vi "runtime execution.vi"() -> (0 "error out":errorcluster)   [LabVIEW 2013, in "Shared Memory Tests.lvlib"]
doc: "Copyright 2016 National Instruments Corporation\n\nLicensed under the Apache License, Version 2.0 (the \"License\"); you may not use this file except in compliance with the License. You may obtain a copy of the License at http://www.apache.org/licenses/LICENSE-2.0\nUnless required by applicable law or agreed to in writing, software distributed under the License is distributed on an \"AS IS\" BASIS, WITHOUT WARRANTIES OR CONDITIONS OF ANY KIND, either express or implied. See the License for the specific language governing permissions and limitations under the License."
uses:
  Shared Memory Tests.lvlib
  module/execution/Shared Memory Runtime.lvclass
  <vilib>/NI/Tag Bus/table/data table.lvlib
  <vilib>/NI/Tag Bus/table/data polymorphs/write many/write Doubles.vi
  <vilib>/NI/Tag Bus/table/data polymorphs/write many/write Booleans.vi
  <vilib>/NI/Tag Bus/table/data polymorphs/write many/write I32s.vi
  <vilib>/NI/Tag Bus/table/data polymorphs/write many/write Singles.vi
  <vilib>/NI/Tag Bus/table/data polymorphs/write many/write I64s.vi
  <vilib>/NI/Tag Bus/table/data polymorphs/write many/write I16s.vi
  <vilib>/NI/Tag Bus/table/data polymorphs/write many/write I8s.vi
  <vilib>/NI/Tag Bus/table/data polymorphs/write many/write U64s.vi
  <vilib>/NI/Tag Bus/table/data polymorphs/write many/write U32s.vi
  <vilib>/NI/Tag Bus/table/data polymorphs/write many/write U16s.vi
  <vilib>/NI/Tag Bus/table/data polymorphs/write many/write U8s.vi
  <vilib>/NI/Tag Bus/table/data polymorphs/write many/write Strings.vi
  module/configuration/Shared Memory Configuration.lvclass
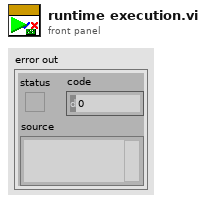
[diagram p1: front panel]
types:
  T1 = typedef "TBM channel.lvclass/data tables.ctl" = cluster{"input data":T2, "processing parameter":T2, "processing result":T2, "output data":T2}
  T2 = typedef "tag bus.lvlib/dictionary table pair.ctl" = cluster{"data dictionary":refnum<class "data dictionary.lvclass">, "data table":T3}
  T3 = typedef "tag bus.lvlib/data table.lvlib/data table.ctl" = cluster{"Double":dbl[], "Single":sgl[], "I64":i64[], "I32":i32[], "I16":i16[], "I8":i8[], "U64":u64[], "U32":u32[], "U16":u16[], "U8":u8[], "Boolean":bool[], "String":string[], "Array of Double":cluster{"DBL Array":dbl[]}[], "Array of Single":cluster{"SGL Array":sgl[]}[], "Array of I64":cluster{"I64 Array":i64[]}[], "Array of I32":cluster{"I32 Array":i32[]}[], "Array of I16":cluster{"I16 Array":i16[]}[], "Array of I8":cluster{"I8 Array":i8[]}[], "Array of U64":cluster{"U64 Array":u64[]}[], "Array of U32":cluster{"U32 Array":u32[]}[], "Array of U16":cluster{"U16 Array":u16[]}[], "Array of U8":cluster{"U8 Array":u8[]}[], "Array of Boolean":cluster{"Boolean Array":bool[]}[], "Array of String":cluster{"String Array":string[]}[]}
  T4 = typedef "current tag file io module runtime.lvclass/current tag file io configuration.ctl" = cluster{"refnum":refnum<file>, "name":string, "data type":T5, "number of tags":i32, "indices":cluster{"index":i32[]}, "data array":cluster{"data":dbl[]}, "file array":cluster{"data":dbl[]}}
  T5 = typedef "tag bus.lvlib/tag descriptor.lvclass/Data Type.ctl" = enum16{"Double", "Single", "I64", "I32", "I16", "I8", "U64", "U32", "U16", "U8", "Boolean", "String", "Array of Double", "Array of Single", "Array of I64", "Array of I32", "Array of I16", "Array of I8", "Array of U64", "Array of U32", "Array of U16", "Array of U8", "Array of Boolean", "Array of String"}
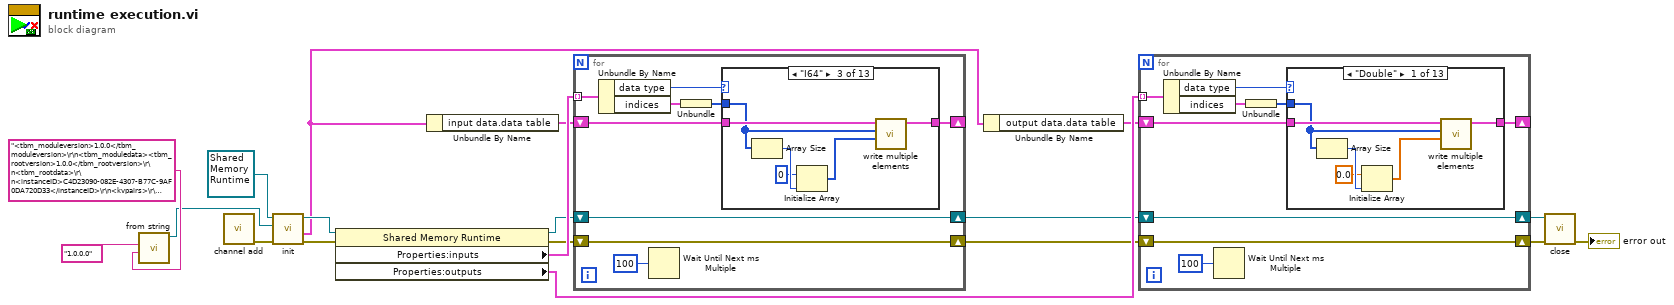
[diagram p0: block diagram]
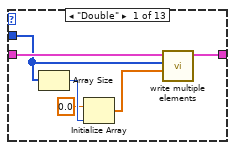
[diagram p2: hidden frame]
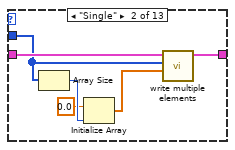
[diagram p3: hidden frame]
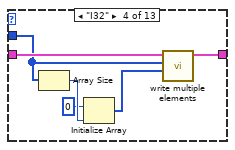
[diagram p4: hidden frame]
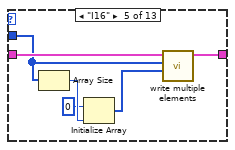
[diagram p5: hidden frame]
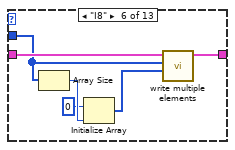
[diagram p6: hidden frame]
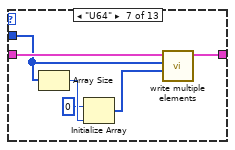
[diagram p7: hidden frame]
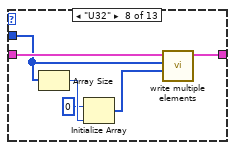
[diagram p8: hidden frame]
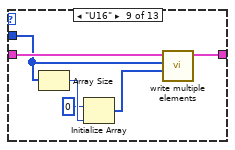
[diagram p9: hidden frame]
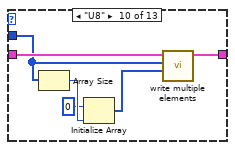
[diagram p10: hidden frame]
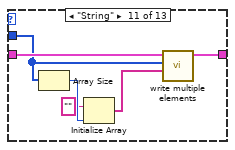
[diagram p11: hidden frame]
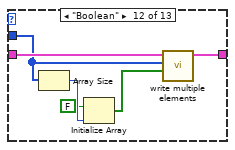
[diagram p12: hidden frame]
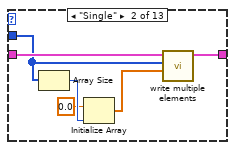
[diagram p14: hidden frame]
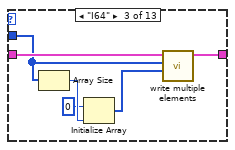
[diagram p15: hidden frame]
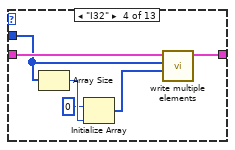
[diagram p16: hidden frame]
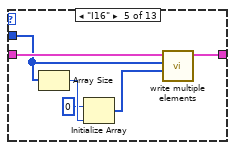
[diagram p17: hidden frame]
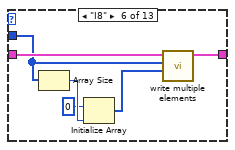
[diagram p18: hidden frame]
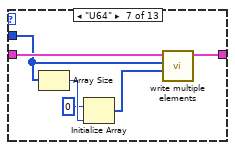
[diagram p19: hidden frame]
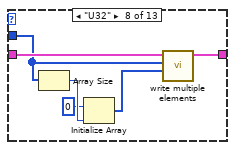
[diagram p20: hidden frame]
diagram:
  n1 = call-dynamic "from string.vi"("data"="<tbm_moduleversion>1.0.0</tbm_moduleversion>\r\n<tbm_moduledata><tbm_rootversion>1.0.0</tbm_rootversion>\r\n<tbm_rootdata>\r\n<instanceID>C4D23090-082E-4307-B77C-9AF0DA720D33</instanceID>\r\n<kvpairs>\r\n<SCFG_AliasName>Shared Memory</SCFG_AliasName>\r\n</kvpairs>\r\n</tbm_rootdata></tbm_moduledata>\r\n<Shared Memory><Cluster>\r\n<Name>shared memory configuration</Name>\r\n<NumElts>3</NumElts>\r\n<Array>\r\n<Name>lines</Name>\r\n<Dimsize>30</Dimsize>\r\n<Cluster>\r\n<Name>alarm config</Name>\r\n<NumElts>3</NumElts>\r\n<String>\r\n<Name>name</Name>\r\n<Val>AI0</Val>\r\n</String>\r\n<EW>\r\n<Name>data type</Name>\r\n<Choice>Double</Choice>\r\n<Choice>Single</Choice>\r\n<Choice>I64</Choice>\r\n<Choice>I32</Choice>\r\n<Choice>I16</Choice>\r\n<Choice>I8</Choice>\r\n<Choice>U64</Choice>\r\n<Choice>U32</Choice>\r\n<Choice>U16</Choice>\r\n<Choice>U8</Choice>\r\n<Choice>Boolean</Choice>\r\n<Choice>String</Choice>\r\n<Choice>Array of Double</Choice>\r\n<Choice>Array of Single</Choice>\r\n<Choice>Array of I64</Choice>\r\n<Choice>Array of I32</Choice>\r\n<Choice>Array of I16</Choice>\r\n<Choice>Array of I8</Choice>\r\n<Choice>Array of U64</Choice>\r\n<Choice>Array of U32</Choice>\r\n<Choice>Array of U16</Choice>\r\n<Choice>Array of U8</Choice>\r\n<Choice>Array of Boolean</Choice>\r\n<Choice>Array of String</Choice>\r\n<Val>0</Val>\r\n</EW>\r\n<Object>\r\n<Name>channel</Name>\r\n<NumLevels>2</NumLevels>\r\n<Class>TBM channel.lvclass</Class>\r\n<Version>1.0.0.3</Version>\r\n<Version>1.0.0.4</Version>\r\n<Cluster>\r\n<Name>tag descriptor.lvclass</Name>\r\n<NumElts>4</NumElts>\r\n<String>\r\n<Name>name</Name>\r\n<Val>AI0</Val>\r\n</String>\r\n<EW>\r\n<Name>data type</Name>\r\n<Choice>Double</Choice>\r\n<Choice>Single</Choice>\r\n<Choice>I64</Choice>\r\n<Choice>I32</Choice>\r\n<Choice>I16</Choice>\r\n<Choice>I8</Choice>\r\n<Choice>U64</Choice>\r\n<Choice>U32</Choice>\r\n<Choice>U16</Choice>\r\n<Choice>U8</Choice>\r\n<Choice>Boolean</Choice>\r\n<Choice>String</Choice>\r\n<Choice>Array of Double</Choice>\r\n<Choice>Array of Single</Choice>\r\n<Choice>Array of I64</Choice>\r\n<Choice>Array of I32</Choice>\r\n<Choice>Array of I16</Choice>\r\n<Choice>Array of I8</Choice>\r\n<Choice>Array of U64</Choice>\r\n<Choice>Array of U32</Choice>\r\n<Choice>Array of U16</Choice>\r\n<Choice>Array of U8</Choice>\r\n<Choice>Array of Boolean</Choice>\r\n<Choice>Array of String</Choice>\r\n<Val>0</Val>\r\n</EW>\r\n<String>\r\n<Name>default</Name>\r\n<Val></Val>\r\n</String>\r\n<String>\r\n<Name>metadata</Name>\r\n<Val></Val>\r\n</String>\r\n</Cluster>\r\n<Cluster>\r\n<Name>TBM channel.lvclass</Name>\r\n<NumElts>1</NumElts>\r\n<EW>\r\n<Name>channel classification</Name>\r\n<Choice>input data</Choice>\r\n<Choice>output data</Choice>\r\n<Choice>processing parameter</Choice>\r\n<Choice>processing result</Choice>\r\n<Val>1</Val>\r\n</EW>\r\n</Cluster>\r\n</Object>\r\n</Cluster>\r\n<Cluster>\r\n<Name>alarm config</Name>\r\n<NumElts>3</NumElts>\r\n<String>\r\n<Name>name</Name>\r\n<Val>AI1</Val>\r\n</String>\r\n<EW>\r\n<Name>data type</Name>\r\n<Choice>Double</Choice>\r\n<Choice>Single</Choice>\r\n<Choice>I64</Choice>\r\n<Choice>I32</Choice>\r\n<Choice>I16</Choice>\r\n<Choice>I8</Choice>\r\n<Choice>U64</Choice>\r\n<Choice>U32</Choice>\r\n<Choice>U16</Choice>\r\n<Choice>U8</Choice>\r\n<Choice>Boolean</Choice>\r\n<Choice>String</Choice>\r\n<Choice>Array of Double</Choice>\r\n<Choice>Array of Single</Choice>\r\n<Choice>Array of I64</Choice>\r\n<Choice>Array of I32</Choice>\r\n<Choice>Array of I16</Choice>\r\n<Choice>Array of I8</Choice>\r\n<Choice>Array of U64</Choice>\r\n<Choice>Array of U32</Choice>\r\n<Choice>Array of U16</Choice>\r\n<Choice>Array of U8</Choice>\r\n<Choice>Array of Boolean</Choice>\r\n<Choice>Array of String</Choice>\r\n<Val>10</Val>\r\n</EW>\r\n<Object>\r\n<Name>channel</Name>\r\n<NumLevels>2</NumLevels>\r\n<Class>TBM channel.lvclass</Class>\r\n<Version>1.0.0.3</Version>\r\n<Version>1.0.0.4</Version>\r\n<Cluster>\r\n<Name>tag descriptor.lvclass</Name>\r\n<NumElts>4</NumElts>\r\n<String>\r\n<Name>name</Name>\r\n<Val>AI1</Val>\r\n</String>\r\n<EW>\r\n<Name>data type</Name>\r\n<Choice>Double</Choice>\r\n<Choice>Single</Choice>\r\n<Choice>I64</Choice>\r\n<Choice>I32</Choice>\r\n<Choice>I16</Choice>\r\n<Choice>I8</Choice>\r\n<Choice>U64</Choice>\r\n<Choice>U32</Choice>\r\n<Choice>U16</Choice>\r\n<Choice>U8</Choice>\r\n<Choice>Boolean</Choice>\r\n<Choice>String</Choice>\r\n<Choice>Array of Double</Choice>\r\n<Choice>Array of Single</Choice>\r\n<Choice>Array of I64</Choice>\r\n<Choice>Array of I32</Choice>\r\n<Choice>Array of I16</Choice>\r\n<Choice>Array of I8</Choice>\r\n<Choice>Array of U64</Choice>\r\n<Choice>Array of U32</Choice>\r\n<Choice>Array of U16</Choice>\r\n<Choice>Array of U8</Choice>\r\n<Choice>Array of Boolean</Choice>\r\n<Choice>Array of String</Choice>\r\n<Val>10</Val>\r\n</EW>\r\n<String>\r\n<Name>default</Name>\r\n<Val></Val>\r\n</String>\r\n<String>\r\n<Name>metadata</Name>\r\n<Val></Val>\r\n</String>\r\n</Cluster>\r\n<Cluster>\r\n<Name>TBM channel.lvclass</Name>\r\n<NumElts>1</NumElts>\r\n<EW>\r\n<Name>channel classification</Name>\r\n<Choice>input data</Choice>\r\n<Choice>output data</Choice>\r\n<Choice>processing parameter</Choice>\r\n<Choice>processing result</Choice>\r\n<Val>1</Val>\r\n</EW>\r\n</Cluster>\r\n</Object>\r\n</Cluster>\r\n<Cluster>\r\n<Name>alarm config</Name>\r\n<NumElts>3</NumElts>\r\n<String>\r\n<Name>name</Name>\r\n<Val>AI2</Val>\r\n</String>\r\n<EW>\r\n<Name>data type</Name>\r\n<Choice>Double</Choice>\r\n<Choice>Single</Choice>\r\n<Choice>I64</Choice>\r\n<Choice>I32</Choice>\r\n<Choice>I16</Choice>\r\n<Choice>I8</Choice>\r\n<Choice>U64</Choice>\r\n<Choice>U32</Choice>\r\n<Choice>U16</Choice>\r\n<Choice>U8</Choice>\r\n<Choice>Boolean</Choice>\r\n<Choice>String</Choice>\r\n<Choice>Array of Double</Choice>\r\n<Choice>Array of Single</Choice>\r\n<Choice>Array of I64</Choice>\r\n<Choice>Array of I32</Choice>\r\n<Choice>Array of I16</Choice>\r\n<Choice>Array of I8</Choice>\r\n<Choice>Array of U64</Choice>\r\n<Choice>Array of U32</Choice>\r\n<Choice>Array of U16</Choice>\r\n<Choice>Array of U8</Choice>\r\n<Choice>Array of Boolean</Choice>\r\n<Choice>Array of String</Choice>\r\n<Val>3</Val>\r\n</EW>\r\n<Object>\r\n<Name>channel</Name>\r\n<NumLevels>2</NumLevels>\r\n<Class>TBM channel.lvclass</Class>\r\n<Version>1.0.0.3</Version>\r\n<Version>1.0.0.4</Version>\r\n<Cluster>\r\n<Name>tag descriptor.lvclass</Name>\r\n<NumElts>4</NumElts>\r\n<String>\r\n<Name>name</Name>\r\n<Val>AI2</Val>\r\n</String>\r\n<EW>\r\n<Name>data type</Name>\r\n<Choice>Double</Choice>\r\n<Choice>Single</Choice>\r\n<Choice>I64</Choice>\r\n<Choice>I32</Choice>\r\n<Choice>I16</Choice>\r\n<Choice>I8</Choice>\r\n<Choice>U64</Choice>\r\n<Choice>U32</Choice>\r\n<Choice>U16</Choice>\r\n<Choice>U8</Choice>\r\n<Choice>Boolean</Choice>\r\n<Choice>String</Choice>\r\n<Choice>Array of Double</Choice>\r\n<Choice>Array of Single</Choice>\r\n<Choice>Array of I64</Choice>\r\n<Choice>Array of I32</Choice>\r\n<Choice>Array of I16</Choice>\r\n<Choice>Array of I8</Choice>\r\n<Choice>Array of U64</Choice>\r\n<Choice>Array of U32</Choice>\r\n<Choice>Array of U16</Choice>\r\n<Choice>Array of U8</Choice>\r\n<Choice>Array of Boolean</Choice>\r\n<Choice>Array of String</Choice>\r\n<Val>3</Val>\r\n</EW>\r\n<String>\r\n<Name>default</Name>\r\n<Val></Val>\r\n</String>\r\n<String>\r\n<Name>metadata</Name>\r\n<Val></Val>\r\n</String>\r\n</Cluster>\r\n<Cluster>\r\n<Name>TBM channel.lvclass</Name>\r\n<NumElts>1</NumElts>\r\n<EW>\r\n<Name>channel classification</Name>\r\n<Choice>input data</Choice>\r\n<Choice>output data</Choice>\r\n<Choice>processing parameter</Choice>\r\n<Choice>processing result</Choice>\r\n<Val>1</Val>\r\n</EW>\r\n</Cluster>\r\n</Object>\r\n</Cluster>\r\n<Cluster>\r\n<Name>alarm config</Name>\r\n<NumElts>3</NumElts>\r\n<String>\r\n<Name>name</Name>\r\n<Val>AI3</Val>\r\n</String>\r\n<EW>\r\n<Name>data type</Name>\r\n<Choice>Double</Choice>\r\n<Choice>Single</Choice>\r\n<Choice>I64</Choice>\r\n<Choice>I32</Choice>\r\n<Choice>I16</Choice>\r\n<Choice>I8</Choice>\r\n<Choice>U64</Choice>\r\n<Choice>U32</Choice>\r\n<Choice>U16</Choice>\r\n<Choice>U8</Choice>\r\n<Choice>Boolean</Choice>\r\n<Choice>String</Choice>\r\n<Choice>Array of Double</Choice>\r\n<Choice>Array of Single</Choice>\r\n<Choice>Array of I64</Choice>\r\n<Choice>Array of I32</Choice>\r\n<Choice>Array of I16</Choice>\r\n<Choice>Array of I8</Choice>\r\n<Choice>Array of U64</Choice>\r\n<Choice>Array of U32</Choice>\r\n<Choice>Array of U16</Choice>\r\n<Choice>Array of U8</Choice>\r\n<Choice>Array of Boolean</Choice>\r\n<Choice>Array of String</Choice>\r\n<Val>0</Val>\r\n</EW>\r\n<Object>\r\n<Name>channel</Name>\r\n<NumLevels>2</NumLevels>\r\n<Class>TBM channel.lvclass</Class>\r\n<Version>1.0.0.3</Version>\r\n<Version>1.0.0.4</Version>\r\n<Cluster>\r\n<Name>tag descriptor.lvclass</Name>\r\n<NumElts>4</NumElts>\r\n<String>\r\n<Name>name</Name>\r\n<Val>AI3</Val>\r\n</String>\r\n<EW>\r\n<Name>data type</Name>\r\n<Choice>Double</Choice>\r\n<Choice>Single</Choice>\r\n<Choice>I64</Choice>\r\n<Choice>I32</Choice>\r\n<Choice>I16</Choice>\r\n<Choice>I8</Choice>\r\n<Choice>U64</Choice>\r\n<Choice>U32</Choice>\r\n<Choice>U16</Choice>\r\n<Choice>U8</Choice>\r\n<Choice>Boolean</Choice>\r\n<Choice>String</Choice>\r\n<Choice>Array of Double</Choice>\r\n<Choice>Array of Single</Choice>\r\n<Choice>Array of I64</Choice>\r\n<Choice>Array of I32</Choice>\r\n<Choice>Array of I16</Choice>\r\n<Choice>Array of I8</Choice>\r\n<Choice>Array of U64</Choice>\r\n<Choice>Array of U32</Choice>\r\n<Choice>Array of U16</Choice>\r\n<Choice>Array of U8</Choice>\r\n<Choice>Array of Boolean</Choice>\r\n<Choice>Array of String</Choice>\r\n<Val>0</Val>\r\n</EW>\r\n<String>\r\n<Name>default</Name>\r\n<Val></Val>\r\n</String>\r\n<String>\r\n<Name>metadata</Name>\r\n<Val></Val>\r\n</String>\r\n</Cluster>\r\n<Cluster>\r\n<Name>TBM channel.lvclass</Name>\r\n<NumElts>1</NumElts>\r\n<EW>\r\n<Name>channel classification</Name>\r\n<Choice>input data</Choice>\r\n<Choice>output data</Choice>\r\n<Choice>processing parameter</Choice>\r\n<Choice>processing result</Choice>\r\n<Val>1</Val>\r\n</EW>\r\n</Cluster>\r\n</Object>\r\n</Cluster>\r\n<Cluster>\r\n<Name>alarm config</Name>\r\n<NumElts>3</NumElts>\r\n<String>\r\n<Name>name</Name>\r\n<Val>AI4</Val>\r\n</String>\r\n<EW>\r\n<Name>data type</Name>\r\n<Choice>Double</Choice>\r\n<Choice>Single</Choice>\r\n<Choice>I64</Choice>\r\n<Choice>I32</Choice>\r\n<Choice>I16</Choice>\r\n<Choice>I8</Choice>\r\n<Choice>U64</Choice>\r\n<Choice>U32</Choice>\r\n<Choice>U16</Choice>\r\n<Choice>U8</Choice>\r\n<Choice>Boolean</Choice>\r\n<Choice>String</Choice>\r\n<Choice>Array of Double</Choice>\r\n<Choice>Array of Single</Choice>\r\n<Choice>Array of I64</Choice>\r\n<Choice>Array of I32</Choice>\r\n<Choice>Array of I16</Choice>\r\n<Choice>Array of I8</Choice>\r\n<Choice>Array of U64</Choice>\r\n<Choice>Array of U32</Choice>\r\n<Choice>Array of U16</Choice>\r\n<Choice>Array of U8</Choice>\r\n<Choice>Array of Boolean</Choice>\r\n<Choice>Array of String</Choice>\r\n<Val>10</Val>\r\n</EW>\r\n<Object>\r\n<Name>channel</Name>\r\n<NumLevels>2</NumLevels>\r\n<Class>TBM channel.lvclass</Class>\r\n<Version>1.0.0.3</Version>\r\n<Version>1.0.0.4</Version>\r\n<Cluster>\r\n<Name>tag descriptor.lvclass</Name>\r\n<NumElts>4</NumElts>\r\n<String>\r\n<Name>name</Name>\r\n<Val>AI4</Val>\r\n</String>\r\n<EW>\r\n<Name>data type</Name>\r\n<Choice>Double</Choice>\r\n<Choice>Single</Choice>\r\n<Choice>I64</Choice>\r\n<Choice>I32</Choice>\r\n<Choice>I16</Choice>\r\n<Choice>I8</Choice>\r\n<Choice>U64</Choice>\r\n<Choice>U32</Choice>\r\n<Choice>U16</Choice>\r\n<Choice>U8</Choice>\r\n<Choice>Boolean</Choice>\r\n<Choice>String</Choice>\r\n<Choice>Array of Double</Choice>\r\n<Choice>Array of Single</Choice>\r\n<Choice>Array of I64</Choice>\r\n<Choice>Array of I32</Choice>\r\n<Choice>Array of I16</Choice>\r\n<Choice>Array of I8</Choice>\r\n<Choice>Array of U64</Choice>\r\n<Choice>Array of U32</Choice>\r\n<Choice>Array of U16</Choice>\r\n<Choice>Array of U8</Choice>\r\n<Choice>Array of Boolean</Choice>\r\n<Choice>Array of String</Choice>\r\n<Val>10</Val>\r\n</EW>\r\n<String>\r\n<Name>default</Name>\r\n<Val></Val>\r\n</String>\r\n<String>\r\n<Name>metadata</Name>\r\n<Val></Val>\r\n</String>\r\n</Cluster>\r\n<Cluster>\r\n<Name>TBM channel.lvclass</Name>\r\n<NumElts>1</NumElts>\r\n<EW>\r\n<Name>channel classification</Name>\r\n<Choice>input data</Choice>\r\n<Choice>output data</Choice>\r\n<Choice>processing parameter</Choice>\r\n<Choice>processing result</Choice>\r\n<Val>1</Val>\r\n</EW>\r\n</Cluster>\r\n</Object>\r\n</Cluster>\r\n<Cluster>\r\n<Name>alarm config</Name>\r\n<NumElts>3</NumElts>\r\n<String>\r\n<Name>name</Name>\r\n<Val>AI5</Val>\r\n</String>\r\n<EW>\r\n<Name>data type</Name>\r\n<Choice>Double</Choice>\r\n<Choice>Single</Choice>\r\n<Choice>I64</Choice>\r\n<Choice>I32</Choice>\r\n<Choice>I16</Choice>\r\n<Choice>I8</Choice>\r\n<Choice>U64</Choice>\r\n<Choice>U32</Choice>\r\n<Choice>U16</Choice>\r\n<Choice>U8</Choice>\r\n<Choice>Boolean</Choice>\r\n<Choice>String</Choice>\r\n<Choice>Array of Double</Choice>\r\n<Choice>Array of Single</Choice>\r\n<Choice>Array of I64</Choice>\r\n<Choice>Array of I32</Choice>\r\n<Choice>Array of I16</Choice>\r\n<Choice>Array of I8</Choice>\r\n<Choice>Array of U64</Choice>\r\n<Choice>Array of U32</Choice>\r\n<Choice>Array of U16</Choice>\r\n<Choice>Array of U8</Choice>\r\n<Choice>Array of Boolean</Choice>\r\n<Choice>Array of String</Choice>\r\n<Val>3</Val>\r\n</EW>\r\n<Object>\r\n<Name>channel</Name>\r\n<NumLevels>2</NumLevels>\r\n<Class>TBM channel.lvclass</Class>\r\n<Version>1.0.0.3</Version>\r\n<Version>1.0.0.4</Version>\r\n<Cluster>\r\n<Name>tag descriptor.lvclass</Name>\r\n<NumElts>4</NumElts>\r\n<String>\r\n<Name>name</Name>\r\n<Val>AI5</Val>\r\n</String>\r\n<EW>\r\n<Name>data type</Name>\r\n<Choice>Double</Choice>\r\n<Choice>Single</Choice>\r\n<Choice>I64</Choice>\r\n<Choice>I32</Choice>\r\n<Choice>I16</Choice>\r\n<Choice>I8</Choice>\r\n<Choice>U64</Choice>\r\n<Choice>U32</Choice>\r\n<Choice>U16</Choice>\r\n<Choice>U8</Choice>\r\n<Choice>Boolean</Choice>\r\n<Choice>String</Choice>\r\n<Choice>Array of Double</Choice>\r\n<Choice>Array of Single</Choice>\r\n<Choice>Array of I64</Choice>\r\n<Choice>Array of I32</Choice>\r\n<Choice>Array of I16</Choice>\r\n<Choice>Array of I8</Choice>\r\n<Choice>Array of U64</Choice>\r\n<Choice>Array of U32</Choice>\r\n<Choice>Array of U16</Choice>\r\n<Choice>Array of U8</Choice>\r\n<Choice>Array of Boolean</Choice>\r\n<Choice>Array of String</Choice>\r\n<Val>3</Val>\r\n</EW>\r\n<String>\r\n<Name>default</Name>\r\n<Val></Val>\r\n</String>\r\n<String>\r\n<Name>metadata</Name>\r\n<Val></Val>\r\n</String>\r\n</Cluster>\r\n<Cluster>\r\n<Name>TBM channel.lvclass</Name>\r\n<NumElts>1</NumElts>\r\n<EW>\r\n<Name>channel classification</Name>\r\n<Choice>input data</Choice>\r\n<Choice>output data</Choice>\r\n<Choice>processing parameter</Choice>\r\n<Choice>processing result</Choice>\r\n<Val>1</Val>\r\n</EW>\r\n</Cluster>\r\n</Object>\r\n</Cluster>\r\n<Cluster>\r\n<Name>alarm config</Name>\r\n<NumElts>3</NumElts>\r\n<String>\r\n<Name>name</Name>\r\n<Val>AI6</Val>\r\n</String>\r\n<EW>\r\n<Name>data type</Name>\r\n<Choice>Double</Choice>\r\n<Choice>Single</Choice>\r\n<Choice>I64</Choice>\r\n<Choice>I32</Choice>\r\n<Choice>I16</Choice>\r\n<Choice>I8</Choice>\r\n<Choice>U64</Choice>\r\n<Choice>U32</Choice>\r\n<Choice>U16</Choice>\r\n<Choice>U8</Choice>\r\n<Choice>Boolean</Choice>\r\n<Choice>String</Choice>\r\n<Choice>Array of Double</Choice>\r\n<Choice>Array of Single</Choice>\r\n<Choice>Array of I64</Choice>\r\n<Choice>Array of I32</Choice>\r\n<Choice>Array of I16</Choice>\r\n<Choice>Array of I8</Choice>\r\n<Choice>Array of U64</Choice>\r\n<Choice>Array of U32</Choice>\r\n<Choice>Array of U16</Choice>\r\n<Choice>Array of U8</Choice>\r\n<Choice>Array of Boolean</Choice>\r\n<Choice>Array of String</Choice>\r\n<Val>0</Val>\r\n</EW>\r\n<Object>\r\n<Name>channel</Name>\r\n<NumLevels>2</NumLevels>\r\n<Class>TBM channel.lvclass</Class>\r\n<Version>1.0.0.3</Version>\r\n<Version>1.0.0.4</Version>\r\n<Cluster>\r\n<Name>tag descriptor.lvclass</Name>\r\n<NumElts>4</NumElts>\r\n<String>\r\n<Name>name</Name>\r\n<Val>AI6</Val>\r\n</String>\r\n<EW>\r\n<Name>data type</Name>\r\n<Choice>Double</Choice>\r\n<Choice>Single</Choice>\r\n<Choice>I64</Choice>\r\n<Choice>I32</Choice>\r\n<Choice>I16</Choice>\r\n<Choice>I8</Choice>\r\n<Choice>U64</Choice>\r\n<Choice>U32</Choice>\r\n<Choice>U16</Choice>\r\n<Choice>U8</Choice>\r\n<Choice>Boolean</Choice>\r\n<Choice>String</Choice>\r\n<Choice>Array of Double</Choice>\r\n<Choice>Array of Single</Choice>\r\n<Choice>Array of I64</Choice>\r\n<Choice>Array of I32</Choice>\r\n<Choice>Array of I16</Choice>\r\n<Choice>Array of I8</Choice>\r\n<Choice>Array of U64</Choice>\r\n<Choice>Array of U32</Choice>\r\n<Choice>Array of U16</Choice>\r\n<Choice>Array of U8</Choice>\r\n<Choice>Array of Boolean</Choice>\r\n<Choice>Array of String</Choice>\r\n<Val>0</Val>\r\n</EW>\r\n<String>\r\n<Name>default</Name>\r\n<Val></Val>\r\n</String>\r\n<String>\r\n<Name>metadata</Name>\r\n<Val></Val>\r\n</String>\r\n</Cluster>\r\n<Cluster>\r\n<Name>TBM channel.lvclass</Name>\r\n<NumElts>1</NumElts>\r\n<EW>\r\n<Name>channel classification</Name>\r\n<Choice>input data</Choice>\r\n<Choice>output data</Choice>\r\n<Choice>processing parameter</Choice>\r\n<Choice>processing result</Choice>\r\n<Val>1</Val>\r\n</EW>\r\n</Cluster>\r\n</Object>\r\n</Cluster>\r\n<Cluster>\r\n<Name>alarm config</Name>\r\n<NumElts>3</NumElts>\r\n<String>\r\n<Name>name</Name>\r\n<Val>AI7</Val>\r\n</String>\r\n<EW>\r\n<Name>data type</Name>\r\n<Choice>Double</Choice>\r\n<Choice>Single</Choice>\r\n<Choice>I64</Choice>\r\n<Choice>I32</Choice>\r\n<Choice>I16</Choice>\r\n<Choice>I8</Choice>\r\n<Choice>U64</Choice>\r\n<Choice>U32</Choice>\r\n<Choice>U16</Choice>\r\n<Choice>U8</Choice>\r\n<Choice>Boolean</Choice>\r\n<Choice>String</Choice>\r\n<Choice>Array of Double</Choice>\r\n<Choice>Array of Single</Choice>\r\n<Choice>Array of I64</Choice>\r\n<Choice>Array of I32</Choice>\r\n<Choice>Array of I16</Choice>\r\n<Choice>Array of I8</Choice>\r\n<Choice>Array of U64</Choice>\r\n<Choice>Array of U32</Choice>\r\n<Choice>Array of U16</Choice>\r\n<Choice>Array of U8</Choice>\r\n<Choice>Array of Boolean</Choice>\r\n<Choice>Array of String</Choice>\r\n<Val>10</Val>\r\n</EW>\r\n<Object>\r\n<Name>channel</Name>\r\n<NumLevels>2</NumLevels>\r\n<Class>TBM channel.lvclass</Class>\r\n<Version>1.0.0.3</Version>\r\n<Version>1.0.0.4</Version>\r\n<Cluster>\r\n<Name>tag descriptor.lvclass</Name>\r\n<NumElts>4</NumElts>\r\n<String>\r\n<Name>name</Name>\r\n<Val>AI7</Val>\r\n</String>\r\n<EW>\r\n<Name>data type</Name>\r\n<Choice>Double</Choice>\r\n<Choice>Single</Choice>\r\n<Choice>I64</Choice>\r\n<Choice>I32</Choice>\r\n<Choice>I16</Choice>\r\n<Choice>I8</Choice>\r\n<Choice>U64</Choice>\r\n<Choice>U32</Choice>\r\n<Choice>U16</Choice>\r\n<Choice>U8</Choice>\r\n<Choice>Boolean</Choice>\r\n<Choice>String</Choice>\r\n<Choice>Array of Double</Choice>\r\n<Choice>Array of Single</Choice>\r\n<Choice>Array of I64</Choice>\r\n<Choice>Array of I32</Choice>\r\n<Choice>Array of I16</Choice>\r\n<Choice>Array of I8</Choice>\r\n<Choice>Array of U64</Choice>\r\n<Choice>Array of U32</Choice>\r\n<Choice>Array of U16</Choice>\r\n<Choice>Array of U8</Choice>\r\n<Choice>Array of Boolean</Choice>\r\n<Choice>Array of String</Choice>\r\n<Val>10</Val>\r\n</EW>\r\n<String>\r\n<Name>default</Name>\r\n<Val></Val>\r\n</String>\r\n<String>\r\n<Name>metadata</Name>\r\n<Val></Val>\r\n</String>\r\n</Cluster>\r\n<Cluster>\r\n<Name>TBM channel.lvclass</Name>\r\n<NumElts>1</NumElts>\r\n<EW>\r\n<Name>channel classification</Name>\r\n<Choice>input data</Choice>\r\n<Choice>output data</Choice>\r\n<Choice>processing parameter</Choice>\r\n<Choice>processing result</Choice>\r\n<Val>1</Val>\r\n</EW>\r\n</Cluster>\r\n</Object>\r\n</Cluster>\r\n<Cluster>\r\n<Name>alarm config</Name>\r\n<NumElts>3</NumElts>\r\n<String>\r\n<Name>name</Name>\r\n<Val>AI8</Val>\r\n</String>\r\n<EW>\r\n<Name>data type</Name>\r\n<Choice>Double</Choice>\r\n<Choice>Single</Choice>\r\n<Choice>I64</Choice>\r\n<Choice>I32</Choice>\r\n<Choice>I16</Choice>\r\n<Choice>I8</Choice>\r\n<Choice>U64</Choice>\r\n<Choice>U32</Choice>\r\n<Choice>U16</Choice>\r\n<Choice>U8</Choice>\r\n<Choice>Boolean</Choice>\r\n<Choice>String</Choice>\r\n<Choice>Array of Double</Choice>\r\n<Choice>Array of Single</Choice>\r\n<Choice>Array of I64</Choice>\r\n<Choice>Array of I32</Choice>\r\n<Choice>Array of I16</Choice>\r\n<Choice>Array of I8</Choice>\r\n<Choice>Array of U64</Choice>\r\n<Choice>Array of U32</Choice>\r\n<Choice>Array of U16</Choice>\r\n<Choice>Array of U8</Choice>\r\n<Choice>Array of Boolean</Choice>\r\n<Choice>Array of String</Choice>\r\n<Val>3</Val>\r\n</EW>\r\n<Object>\r\n<Name>channel</Name>\r\n<NumLevels>2</NumLevels>\r\n<Class>TBM channel.lvclass</Class>\r\n<Version>1.0.0.3</Version>\r\n<Version>1.0.0.4</Version>\r\n<Cluster>\r\n<Name>tag descriptor.lvclass</Name>\r\n<NumElts>4</NumElts>\r\n<String>\r\n<Name>name</Name>\r\n<Val>AI8</Val>\r\n</String>\r\n<EW>\r\n<Name>data type</Name>\r\n<Choice>Double</Choice>\r\n<Choice>Single</Choice>\r\n<Choice>I64</Choice>\r\n<Choice>I32</Choice>\r\n<Choice>I16</Choice>\r\n<Choice>I8</Choice>\r\n<Choice>U64</Choice>\r\n<Choice>U32</Choice>\r\n<Choice>U16</Choice>\r\n<Choice>U8</Choice>\r\n<Choice>Boolean</Choice>\r\n<Choice>String</Choice>\r\n<Choice>Array of Double</Choice>\r\n<Choice>Array of Single</Choice>\r\n<Choice>Array of I64</Choice>\r\n<Choice>Array of I32</Choice>\r\n<Choice>Array of I16</Choice>\r\n<Choice>Array of I8</Choice>\r\n<Choice>Array of U64</Choice>\r\n<Choice>Array of U32</Choice>\r\n<Choice>Array of U16</Choice>\r\n<Choice>Array of U8</Choice>\r\n<Choice>Array of Boolean</Choice>\r\n<Choice>Array of String</Choice>\r\n<Val>3</Val>\r\n</EW>\r\n<String>\r\n<Name>default</Name>\r\n<Val></Val>\r\n</String>\r\n<String>\r\n<Name>metadata</Name>\r\n<Val></Val>\r\n</String>\r\n</Cluster>\r\n<Cluster>\r\n<Name>TBM channel.lvclass</Name>\r\n<NumElts>1</NumElts>\r\n<EW>\r\n<Name>channel classification</Name>\r\n<Choice>input data</Choice>\r\n<Choice>output data</Choice>\r\n<Choice>processing parameter</Choice>\r\n<Choice>processing result</Choice>\r\n<Val>1</Val>\r\n</EW>\r\n</Cluster>\r\n</Object>\r\n</Cluster>\r\n<Cluster>\r\n<Name>alarm config</Name>\r\n<NumElts>3</NumElts>\r\n<String>\r\n<Name>name</Name>\r\n<Val>AI9</Val>\r\n</String>\r\n<EW>\r\n<Name>data type</Name>\r\n<Choice>Double</Choice>\r\n<Choice>Single</Choice>\r\n<Choice>I64</Choice>\r\n<Choice>I32</Choice>\r\n<Choice>I16</Choice>\r\n<Choice>I8</Choice>\r\n<Choice>U64</Choice>\r\n<Choice>U32</Choice>\r\n<Choice>U16</Choice>\r\n<Choice>U8</Choice>\r\n<Choice>Boolean</Choice>\r\n<Choice>String</Choice>\r\n<Choice>Array of Double</Choice>\r\n<Choice>Array of Single</Choice>\r\n<Choice>Array of I64</Choice>\r\n<Choice>Array of I32</Choice>\r\n<Choice>Array of I16</Choice>\r\n<Choice>Array of I8</Choice>\r\n<Choice>Array of U64</Choice>\r\n<Choice>Array of U32</Choice>\r\n<Choice>Array of U16</Choice>\r\n<Choice>Array of U8</Choice>\r\n<Choice>Array of Boolean</Choice>\r\n<Choice>Array of String</Choice>\r\n<Val>0</Val>\r\n</EW>\r\n<Object>\r\n<Name>channel</Name>\r\n<NumLevels>2</NumLevels>\r\n<Class>TBM channel.lvclass</Class>\r\n<Version>1.0.0.3</Version>\r\n<Version>1.0.0.4</Version>\r\n<Cluster>\r\n<Name>tag descriptor.lvclass</Name>\r\n<NumElts>4</NumElts>\r\n<String>\r\n<Name>name</Name>\r\n<Val>AI9</Val>\r\n</String>\r\n<EW>\r\n<Name>data type</Name>\r\n<Choice>Double</Choice>\r\n<Choice>Single</Choice>\r\n<Choice>I64</Choice>\r\n<Choice>I32</Choice>\r\n<Choice>I16</Choice>\r\n<Choice>I8</Choice>\r\n<Choice>U64</Choice>\r\n<Choice>U32</Choice>\r\n<Choice>U16</Choice>\r\n<Choice>U8</Choice>\r\n<Choice>Boolean</Choice>\r\n<Choice>String</Choice>\r\n<Choice>Array of Double</Choice>\r\n<Choice>Array of Single</Choice>\r\n<Choice>Array of I64</Choice>\r\n<Choice>Array of I32</Choice>\r\n<Choice>Array of I16</Choice>\r\n<Choice>Array of I8</Choice>\r\n<Choice>Array of U64</Choice>\r\n<Choice>Array of U32</Choice>\r\n<Choice>Array of U16</Choice>\r\n<Choice>Array of U8</Choice>\r\n<Choice>Array of Boolean</Choice>\r\n<Choice>Array of String</Choice>\r\n<Val>0</Val>\r\n</EW>\r\n<String>\r\n<Name>default</Name>\r\n<Val></Val>\r\n</String>\r\n<String>\r\n<Name>metadata</Name>\r\n<Val></Val>\r\n</String>\r\n</Cluster>\r\n<Cluster>\r\n<Name>TBM channel.lvclass</Name>\r\n<NumElts>1</NumElts>\r\n<EW>\r\n<Name>channel classification</Name>\r\n<Choice>input data</Choice>\r\n<Choice>output data</Choice>\r\n<Choice>processing parameter</Choice>\r\n<Choice>processing result</Choice>\r\n<Val>1</Val>\r\n</EW>\r\n</Cluster>\r\n</Object>\r\n</Cluster>\r\n<Cluster>\r\n<Name>alarm config</Name>\r\n<NumElts>3</NumElts>\r\n<String>\r\n<Name>name</Name>\r\n<Val>AO0</Val>\r\n</String>\r\n<EW>\r\n<Name>data type</Name>\r\n<Choice>Double</Choice>\r\n<Choice>Single</Choice>\r\n<Choice>I64</Choice>\r\n<Choice>I32</Choice>\r\n<Choice>I16</Choice>\r\n<Choice>I8</Choice>\r\n<Choice>U64</Choice>\r\n<Choice>U32</Choice>\r\n<Choice>U16</Choice>\r\n<Choice>U8</Choice>\r\n<Choice>Boolean</Choice>\r\n<Choice>String</Choice>\r\n<Choice>Array of Double</Choice>\r\n<Choice>Array of Single</Choice>\r\n<Choice>Array of I64</Choice>\r\n<Choice>Array of I32</Choice>\r\n<Choice>Array of I16</Choice>\r\n<Choice>Array of I8</Choice>\r\n<Choice>Array of U64</Choice>\r\n<Choice>Array of U32</Choice>\r\n<Choice>Array of U16</Choice>\r\n<Choice>Array of U8</Choice>\r\n<Choice>Array of Boolean</Choice>\r\n<Choice>Array of String</Choice>\r\n<Val>10</Val>\r\n</EW>\r\n<Object>\r\n<Name>channel</Name>\r\n<NumLevels>2</NumLevels>\r\n<Class>TBM channel.lvclass</Class>\r\n<Version>1.0.0.3</Version>\r\n<Version>1.0.0.4</Version>\r\n<Cluster>\r\n<Name>tag descriptor.lvclass</Name>\r\n<NumElts>4</NumElts>\r\n<String>\r\n<Name>name</Name>\r\n<Val>AO0</Val>\r\n</String>\r\n<EW>\r\n<Name>data type</Name>\r\n<Choice>Double</Choice>\r\n<Choice>Single</Choice>\r\n<Choice>I64</Choice>\r\n<Choice>I32</Choice>\r\n<Choice>I16</Choice>\r\n<Choice>I8</Choice>\r\n<Choice>U64</Choice>\r\n<Choice>U32</Choice>\r\n<Choice>U16</Choice>\r\n<Choice>U8</Choice>\r\n<Choice>Boolean</Choice>\r\n<Choice>String</Choice>\r\n<Choice>Array of Double</Choice>\r\n<Choice>Array of Single</Choice>\r\n<Choice>Array of I64</Choice>\r\n<Choice>Array of I32</Choice>\r\n<Choice>Array of I16</Choice>\r\n<Choice>Array of I8</Choice>\r\n<Choice>Array of U64</Choice>\r\n<Choice>Array of U32</Choice>\r\n<Choice>Array of U16</Choice>\r\n<Choice>Array of U8</Choice>\r\n<Choice>Array of Boolean</Choice>\r\n<Choice>Array of String</Choice>\r\n<Val>10</Val>\r\n</EW>\r\n<String>\r\n<Name>default</Name>\r\n<Val></Val>\r\n</String>\r\n<String>\r\n<Name>metadata</Name>\r\n<Val></Val>\r\n</String>\r\n</Cluster>\r\n<Cluster>\r\n</Cluster>\r\n</Object>\r\n</Cluster>\r\n<Cluster>\r\n<Name>alarm config</Name>\r\n<NumElts>3</NumElts>\r\n<String>\r\n<Name>name</Name>\r\n<Val>AO1</Val>\r\n</String>\r\n<EW>\r\n<Name>data type</Name>\r\n<Choice>Double</Choice>\r\n<Choice>Single</Choice>\r\n<Choice>I64</Choice>\r\n<Choice>I32</Choice>\r\n<Choice>I16</Choice>\r\n<Choice>I8</Choice>\r\n<Choice>U64</Choice>\r\n<Choice>U32</Choice>\r\n<Choice>U16</Choice>\r\n<Choice>U8</Choice>\r\n<Choice>Boolean</Choice>\r\n<Choice>String</Choice>\r\n<Choice>Array of Double</Choice>\r\n<Choice>Array of Single</Choice>\r\n<Choice>Array of I64</Choice>\r\n<Choice>Array of I32</Choice>\r\n<Choice>Array of I16</Choice>\r\n<Choice>Array of I8</Choice>\r\n<Choice>Array of U64</Choice>\r\n<Choice>Array of U32</Choice>\r\n<Choice>Array of U16</Choice>\r\n<Choice>Array of U8</Choice>\r\n<Choice>Array of Boolean</Choice>\r\n<Choice>Array of String</Choice>\r\n<Val>3</Val>\r\n</EW>\r\n<Object>\r\n<Name>channel</Name>\r\n<NumLevels>2</NumLevels>\r\n<Class>TBM channel.lvclass</Class>\r\n<Version>1.0.0.3</Version>\r\n<Version>1.0.0.4</Version>\r\n<Cluster>\r\n<Name>tag descriptor.lvclass</Name>\r\n<NumElts>4</NumElts>\r\n<String>\r\n<Name>name</Name>\r\n<Val>AO1</Val>\r\n</String>\r\n<EW>\r\n<Name>data type</Name>\r\n<Choice>Double</Choice>\r\n<Choice>Single</Choice>\r\n<Choice>I64</Choice>\r\n<Choice>I32</Choice>\r\n<Choice>I16</Choice>\r\n<Choice>I8</Choice>\r\n<Choice>U64</Choice>\r\n<Choice>U32</Choice>\r\n<Choice>U16</Choice>\r\n<Choice>U8</Choice>\r\n<Choice>Boolean</Choice>\r\n<Choice>String</Choice>\r\n<Choice>Array of Double</Choice>\r\n<Choice>Array of Single</Choice>\r\n<Choice>Array of I64</Choice>\r\n<Choice>Array of I32</Choice>\r\n<Choice>Array of I16</Choice>\r\n<Choice>Array of I8</Choice>\r\n<Choice>Array of U64</Choice>\r\n<Choice>Array of U32</Choice>\r\n<Choice>Array of U16</Choice>\r\n<Choice>Array of U8</Choice>\r\n<Choice>Array of Boolean</Choice>\r\n<Choice>Array of String</Choice>\r\n<Val>3</Val>\r\n</EW>\r\n<String>\r\n<Name>default</Name>\r\n<Val></Val>\r\n</String>\r\n<String>\r\n<Name>metadata</Name>\r\n<Val></Val>\r\n</String>\r\n</Cluster>\r\n<Cluster>\r\n</Cluster>\r\n</Object>\r\n</Cluster>\r\n<Cluster>\r\n<Name>alarm config</Name>\r\n<NumElts>3</NumElts>\r\n<String>\r\n<Name>name</Name>\r\n<Val>AO2</Val>\r\n</String>\r\n<EW>\r\n<Name>data type</Name>\r\n<Choice>Double</Choice>\r\n<Choice>Single</Choice>\r\n<Choice>I64</Choice>\r\n<Choice>I32</Choice>\r\n<Choice>I16</Choice>\r\n<Choice>I8</Choice>\r\n<Choice>U64</Choice>\r\n<Choice>U32</Choice>\r\n<Choice>U16</Choice>\r\n<Choice>U8</Choice>\r\n<Choice>Boolean</Choice>\r\n<Choice>String</Choice>\r\n<Choice>Array of Double</Choice>\r\n<Choice>Array of Single</Choice>\r\n<Choice>Array of I64</Choice>\r\n<Choice>Array of I32</Choice>\r\n<Choice>Array of I16</Choice>\r\n<Choice>Array of I8</Choice>\r\n<Choice>Array of U64</Choice>\r\n<Choice>Array of U32</Choice>\r\n<Choice>Array of U16</Choice>\r\n<Choice>Array of U8</Choice>\r\n<Choice>Array of Boolean</Choice>\r\n<Choice>Array of String</Choice>\r\n<Val>0</Val>\r\n</EW>\r\n<Object>\r\n<Name>channel</Name>\r\n<NumLevels>2</NumLevels>\r\n<Class>TBM channel.lvclass</Class>\r\n<Version>1.0.0.3</Version>\r\n<Version>1.0.0.4</Version>\r\n<Cluster>\r\n<Name>tag descriptor.lvclass</Name>\r\n<NumElts>4</NumElts>\r\n<String>\r\n<Name>name</Name>\r\n<Val>AO2</Val>\r\n</String>\r\n<EW>\r\n<Name>data type</Name>\r\n<Choice>Double</Choice>\r\n<Choice>Single</Choice>\r\n<Choice>I64</Choice>\r\n<Choice>I32</Choice>\r\n<Choice>I16</Choice>\r\n<Choice>I8</Choice>\r\n<Choice>U64</Choice>\r\n<Choice>U32</Choice>\r\n<Choice>U16</Choice>\r\n<Choice>U8</Choice>\r\n<Choice>Boolean</Choice>\r\n<Choice>String</Choice>\r\n<Choice>Array of Double</Choice>\r\n<Choice>Array of Single</Choice>\r\n<Choice>Array of I64</Choice>\r\n<Choice>Array of I32</Choice>\r\n<Choice>Array of I16</Choice>\r\n<Choice>Array of I8</Choice>\r\n<Choice>Array of U64</Choice>\r\n<Choice>Array of U32</Choice>\r\n<Choice>Array of U16</Choice>\r\n<Choice>Array of U8</Choice>\r\n<Choice>Array of Boolean</Choice>\r\n<Choice>Array of String</Choice>\r\n<Val>0</Val>\r\n</EW>\r\n<String>\r\n<Name>default</Name>\r\n<Val></Val>\r\n</String>\r\n<String>\r\n<Name>metadata</Name>\r\n<Val></Val>\r\n</String>\r\n</Cluster>\r\n<Cluster>\r\n</Cluster>\r\n</Object>\r\n</Cluster>\r\n<Cluster>\r\n<Name>alarm config</Name>\r\n<NumElts>3</NumElts>\r\n<String>\r\n<Name>name</Name>\r\n<Val>AO3</Val>\r\n</String>\r\n<EW>\r\n<Name>data type</Name>\r\n<Choice>Double</Choice>\r\n<Choice>Single</Choice>\r\n<Choice>I64</Choice>\r\n<Choice>I32</Choice>\r\n<Choice>I16</Choice>\r\n<Choice>I8</Choice>\r\n<Choice>U64</Choice>\r\n<Choice>U32</Choice>\r\n<Choice>U16</Choice>\r\n<Choice>U8</Choice>\r\n<Choice>Boolean</Choice>\r\n<Choice>String</Choice>\r\n<Choice>Array of Double</Choice>\r\n<Choice>Array of Single</Choice>\r\n<Choice>Array of I64</Choice>\r\n<Choice>Array of I32</Choice>\r\n<Choice>Array of I16</Choice>\r\n<Choice>Array of I8</Choice>\r\n<Choice>Array of U64</Choice>\r\n<Choice>Array of U32</Choice>\r\n<Choice>Array of U16</Choice>\r\n<Choice>Array of U8</Choice>\r\n<Choice>Array of Boolean</Choice>\r\n<Choice>Array of String</Choice>\r\n<Val>10</Val>\r\n</EW>\r\n<Object>\r\n<Name>channel</Name>\r\n<NumLevels>2</NumLevels>\r\n<Class>TBM channel.lvclass</Class>\r\n<Version>1.0.0.3</Version>\r\n<Version>1.0.0.4</Version>\r\n<Cluster>\r\n<Name>tag descriptor.lvclass</Name>\r\n<NumElts>4</NumElts>\r\n<String>\r\n<Name>name</Name>\r\n<Val>AO3</Val>\r\n</String>\r\n<EW>\r\n<Name>data type</Name>\r\n<Choice>Double</Choice>\r\n<Choice>Single</Choice>\r\n<Choice>I64</Choice>\r\n<Choice>I32</Choice>\r\n<Choice>I16</Choice>\r\n<Choice>I8</Choice>\r\n<Choice>U64</Choice>\r\n<Choice>U32</Choice>\r\n<Choice>U16</Choice>\r\n<Choice>U8</Choice>\r\n<Choice>Boolean</Choice>\r\n<Choice>String</Choice>\r\n<Choice>Array of Double</Choice>\r\n<Choice>Array of Single</Choice>\r\n<Choice>Array of I64</Choice>\r\n<Choice>Array of I32</Choice>\r\n<Choice>Array of I16</Choice>\r\n<Choice>Array of I8</Choice>\r\n<Choice>Array of U64</Choice>\r\n<Choice>Array of U32</Choice>\r\n<Choice>Array of U16</Choice>\r\n<Choice>Array of U8</Choice>\r\n<Choice>Array of Boolean</Choice>\r\n<Choice>Array of String</Choice>\r\n<Val>10</Val>\r\n</EW>\r\n<String>\r\n<Name>default</Name>\r\n<Val></Val>\r\n</String>\r\n<String>\r\n<Name>metadata</Name>\r\n<Val></Val>\r\n</String>\r\n</Cluster>\r\n<Cluster>\r\n</Cluster>\r\n</Object>\r\n</Cluster>\r\n<Cluster>\r\n<Name>alarm config</Name>\r\n<NumElts>3</NumElts>\r\n<String>\r\n<Name>name</Name>\r\n<Val>AO4</Val>\r\n</String>\r\n<EW>\r\n<Name>data type</Name>\r\n<Choice>Double</Choice>\r\n<Choice>Single</Choice>\r\n<Choice>I64</Choice>\r\n<Choice>I32</Choice>\r\n<Choice>I16</Choice>\r\n<Choice>I8</Choice>\r\n<Choice>U64</Choice>\r\n<Choice>U32</Choice>\r\n<Choice>U16</Choice>\r\n<Choice>U8</Choice>\r\n<Choice>Boolean</Choice>\r\n<Choice>String</Choice>\r\n<Choice>Array of Double</Choice>\r\n<Choice>Array of Single</Choice>\r\n<Choice>Array of I64</Choice>\r\n<Choice>Array of I32</Choice>\r\n<Choice>Array of I16</Choice>\r\n<Choice>Array of I8</Choice>\r\n<Choice>Array of U64</Choice>\r\n<Choice>Array of U32</Choice>\r\n<Choice>Array of U16</Choice>\r\n<Choice>Array of U8</Choice>\r\n<Choice>Array of Boolean</Choice>\r\n<Choice>Array of String</Choice>\r\n<Val>3</Val>\r\n</EW>\r\n<Object>\r\n<Name>channel</Name>\r\n<NumLevels>2</NumLevels>\r\n<Class>TBM channel.lvclass</Class>\r\n<Version>1.0.0.3</Version>\r\n<Version>1.0.0.4</Version>\r\n<Cluster>\r\n<Name>tag descriptor.lvclass</Name>\r\n<NumElts>4</NumElts>\r\n<String>\r\n<Name>name</Name>\r\n<Val>AO4</Val>\r\n</String>\r\n<EW>\r\n<Name>data type</Name>\r\n<Choice>Double</Choice>\r\n<Choice>Single</Choice>\r\n<Choice>I64</Choice>\r\n<Choice>I32</Choice>\r\n<Choice>I16</Choice>\r\n<Choice>I8</Choice>\r\n<Choice>U64</Choice>\r\n<Choice>U32</Choice>\r\n<Choice>U16</Choice>\r\n<Choice>U8</Choice>\r\n<Choice>Boolean</Choice>\r\n<Choice>String</Choice>\r\n<Choice>Array of Double</Choice>\r\n<Choice>Array of Single</Choice>\r\n<Choice>Array of I64</Choice>\r\n<Choice>Array of I32</Choice>\r\n<Choice>Array of I16</Choice>\r\n<Choice>Array of I8</Choice>\r\n<Choice>Array of U64</Choice>\r\n<Choice>Array of U32</Choice>\r\n<Choice>Array of U16</Choice>\r\n<Choice>Array of U8</Choice>\r\n<Choice>Array of Boolean</Choice>\r\n<Choice>Array of String</Choice>\r\n<Val>3</Val>\r\n</EW>\r\n<String>\r\n<Name>default</Name>\r\n<Val></Val>\r\n</String>\r\n<String>\r\n<Name>metadata</Name>\r\n<Val></Val>\r\n</String>\r\n</Cluster>\r\n<Cluster>\r\n</Cluster>\r\n</Object>\r\n</Cluster>\r\n<Cluster>\r\n<Name>alarm config</Name>\r\n<NumElts>3</NumElts>\r\n<String>\r\n<Name>name</Name>\r\n<Val>AO5</Val>\r\n</String>\r\n<EW>\r\n<Name>data type</Name>\r\n<Choice>Double</Choice>\r\n<Choice>Single</Choice>\r\n<Choice>I64</Choice>\r\n<Choice>I32</Choice>\r\n<Choice>I16</Choice>\r\n<Choice>I8</Choice>\r\n<Choice>U64</Choice>\r\n<Choice>U32</Choice>\r\n<Choice>U16</Choice>\r\n<Choice>U8</Choice>\r\n<Choice>Boolean</Choice>\r\n<Choice>String</Choice>\r\n<Choice>Array of Double</Choice>\r\n<Choice>Array of Single</Choice>\r\n<Choice>Array of I64</Choice>\r\n<Choice>Array of I32</Choice>\r\n<Choice>Array of I16</Choice>\r\n<Choice>Array of I8</Choice>\r\n<Choice>Array of U64</Choice>\r\n<Choice>Array of U32</Choice>\r\n<Choice>Array of U16</Choice>\r\n<Choice>Array of U8</Choice>\r\n<Choice>Array of Boolean</Choice>\r\n<Choice>Array of String</Choice>\r\n<Val>0</Val>\r\n</EW>\r\n<Object>\r\n<Name>channel</Name>\r\n<NumLevels>2</NumLevels>\r\n<Class>TBM channel.lvclass</Class>\r\n<Version>1.0.0.3</Version>\r\n<Version>1.0.0.4</Version>\r\n<Cluster>\r\n<Name>tag descriptor.lvclass</Name>\r\n<NumElts>4</NumElts>\r\n<String>\r\n<Name>name</Name>\r\n<Val>AO5</Val>\r\n</String>\r\n<EW>\r\n<Name>data type</Name>\r\n<Choice>Double</Choice>\r\n<Choice>Single</Choice>\r\n<Choice>I64</Choice>\r\n<Choice>I32</Choice>\r\n<Choice>I16</Choice>\r\n<Choice>I8</Choice>\r\n<Choice>U64</Choice>\r\n<Choice>U32</Choice>\r\n<Choice>U16</Choice>\r\n<Choice>U8</Choice>\r\n<Choice>Boolean</Choice>\r\n<Choice>String</Choice>\r\n<Choice>Array of Double</Choice>\r\n<Choice>Array of Single</Choice>\r\n<Choice>Array of I64</Choice>\r\n<Choice>Array of I32</Choice>\r\n<Choice>Array of I16</Choice>\r\n<Choice>Array of I8</Choice>\r\n<Choice>Array of U64</Choice>\r\n<Choice>Array of U32</Choice>\r\n<Choice>Array of U16</Choice>\r\n<Choice>Array of U8</Choice>\r\n<Choice>Array of Boolean</Choice>\r\n<Choice>Array of String</Choice>\r\n<Val>0</Val>\r\n</EW>\r\n<String>\r\n<Name>default</Name>\r\n<Val></Val>\r\n</String>\r\n<String>\r\n<Name>metadata</Name>\r\n<Val></Val>\r\n</String>\r\n</Cluster>\r\n<Cluster>\r\n</Cluster>\r\n</Object>\r\n</Cluster>\r\n<Cluster>\r\n<Name>alarm config</Name>\r\n<NumElts>3</NumElts>\r\n<String>\r\n<Name>name</Name>\r\n<Val>AO6</Val>\r\n</String>\r\n<EW>\r\n<Name>data type</Name>\r\n<Choice>Double</Choice>\r\n<Choice>Single</Choice>\r\n<Choice>I64</Choice>\r\n<Choice>I32</Choice>\r\n<Choice>I16</Choice>\r\n<Choice>I8</Choice>\r\n<Choice>U64</Choice>\r\n<Choice>U32</Choice>\r\n<Choice>U16</Choice>\r\n<Choice>U8</Choice>\r\n<Choice>Boolean</Choice>\r\n<Choice>String</Choice>\r\n<Choice>Array of Double</Choice>\r\n<Choice>Array of Single</Choice>\r\n<Choice>Array of I64</Choice>\r\n<Choice>Array of I32</Choice>\r\n<Choice>Array of I16</Choice>\r\n<Choice>Array of I8</Choice>\r\n<Choice>Array of U64</Choice>\r\n<Choice>Array of U32</Choice>\r\n<Choice>Array of U16</Choice>\r\n<Choice>Array of U8</Choice>\r\n<Choice>Array of Boolean</Choice>\r\n<Choice>Array of String</Choice>\r\n<Val>10</Val>\r\n</EW>\r\n<Object>\r\n<Name>channel</Name>\r\n<NumLevels>2</NumLevels>\r\n<Class>TBM channel.lvclass</Class>\r\n<Version>1.0.0.3</Version>\r\n<Version>1.0.0.4</Version>\r\n<Cluster>\r\n<Name>tag descriptor.lvclass</Name>\r\n<NumElts>4</NumElts>\r\n<String>\r\n<Name>name</Name>\r\n<Val>AO6</Val>\r\n</String>\r\n<EW>\r\n<Name>data type</Name>\r\n<Choice>Double</Choice>\r\n<Choice>Single</Choice>\r\n<Choice>I64</Choice>\r\n<Choice>I32</Choice>\r\n<Choice>I16</Choice>\r\n<Choice>I8</Choice>\r\n<Choice>U64</Choice>\r\n<Choice>U32</Choice>\r\n<Choice>U16</Choice>\r\n<Choice>U8</Choice>\r\n<Choice>Boolean</Choice>\r\n<Choice>String</Choice>\r\n<Choice>Array of Double</Choice>\r\n<Choice>Array of Single</Choice>\r\n<Choice>Array of I64</Choice>\r\n<Choice>Array of I32</Choice>\r\n<Choice>Array of I16</Choice>\r\n<Choice>Array of I8</Choice>\r\n<Choice>Array of U64</Choice>\r\n<Choice>Array of U32</Choice>\r\n<Choice>Array of U16</Choice>\r\n<Choice>Array of U8</Choice>\r\n<Choice>Array of Boolean</Choice>\r\n<Choice>Array of String</Choice>\r\n<Val>10</Val>\r\n</EW>\r\n<String>\r\n<Name>default</Name>\r\n<Val></Val>\r\n</String>\r\n<String>\r\n<Name>metadata</Name>\r\n<Val></Val>\r\n</String>\r\n</Cluster>\r\n<Cluster>\r\n</Cluster>\r\n</Object>\r\n</Cluster>\r\n<Cluster>\r\n<Name>alarm config</Name>\r\n<NumElts>3</NumElts>\r\n<String>\r\n<Name>name</Name>\r\n<Val>AO7</Val>\r\n</String>\r\n<EW>\r\n<Name>data type</Name>\r\n<Choice>Double</Choice>\r\n<Choice>Single</Choice>\r\n<Choice>I64</Choice>\r\n<Choice>I32</Choice>\r\n<Choice>I16</Choice>\r\n<Choice>I8</Choice>\r\n<Choice>U64</Choice>\r\n<Choice>U32</Choice>\r\n<Choice>U16</Choice>\r\n<Choice>U8</Choice>\r\n<Choice>Boolean</Choice>\r\n<Choice>String</Choice>\r\n<Choice>Array of Double</Choice>\r\n<Choice>Array of Single</Choice>\r\n<Choice>Array of I64</Choice>\r\n<Choice>Array of I32</Choice>\r\n<Choice>Array of I16</Choice>\r\n<Choice>Array of I8</Choice>\r\n<Choice>Array of U64</Choice>\r\n<Choice>Array of U32</Choice>\r\n<Choice>Array of U16</Choice>\r\n<Choice>Array of U8</Choice>\r\n<Choice>Array of Boolean</Choice>\r\n<Choice>Array of String</Choice>\r\n<Val>3</Val>\r\n</EW>\r\n<Object>\r\n<Name>channel</Name>\r\n<NumLevels>2</NumLevels>\r\n<Class>TBM channel.lvclass</Class>\r\n<Version>1.0.0.3</Version>\r\n<Version>1.0.0.4</Version>\r\n<Cluster>\r\n<Name>tag descriptor.lvclass</Name>\r\n<NumElts>4</NumElts>\r\n<String>\r\n<Name>name</Name>\r\n<Val>AO7</Val>\r\n</String>\r\n<EW>\r\n<Name>data type</Name>\r\n<Choice>Double</Choice>\r\n<Choice>Single</Choice>\r\n<Choice>I64</Choice>\r\n<Choice>I32</Choice>\r\n<Choice>I16</Choice>\r\n<Choice>I8</Choice>\r\n<Choice>U64</Choice>\r\n<Choice>U32</Choice>\r\n<Choice>U16</Choice>\r\n<Choice>U8</Choice>\r\n<Choice>Boolean</Choice>\r\n<Choice>String</Choice>\r\n<Choice>Array of Double</Choice>\r\n<Choice>Array of Single</Choice>\r\n<Choice>Array of I64</Choice>\r\n<Choice>Array of I32</Choice>\r\n<Choice>Array of I16</Choice>\r\n<Choice>Array of I8</Choice>\r\n<Choice>Array of U64</Choice>\r\n<Choice>Array of U32</Choice>\r\n<Choice>Array of U16</Choice>\r\n<Choice>Array of U8</Choice>\r\n<Choice>Array of Boolean</Choice>\r\n<Choice>Array of String</Choice>\r\n<Val>3</Val>\r\n</EW>\r\n<String>\r\n<Name>default</Name>\r\n<Val></Val>\r\n</String>\r\n<String>\r\n<Name>metadata</Name>\r\n<Val></Val>\r\n</String>\r\n</Cluster>\r\n<Cluster>\r\n</Cluster>\r\n</Object>\r\n</Cluster>\r\n<Cluster>\r\n<Name>alarm config</Name>\r\n<NumElts>3</NumElts>\r\n<String>\r\n<Name>name</Name>\r\n<Val>AO8</Val>\r\n</String>\r\n<EW>\r\n<Name>data type</Name>\r\n<Choice>Double</Choice>\r\n<Choice>Single</Choice>\r\n<Choice>I64</Choice>\r\n<Choice>I32</Choice>\r\n<Choice>I16</Choice>\r\n<Choice>I8</Choice>\r\n<Choice>U64</Choice>\r\n<Choice>U32</Choice>\r\n<Choice>U16</Choice>\r\n<Choice>U8</Choice>\r\n<Choice>Boolean</Choice>\r\n<Choice>String</Choice>\r\n<Choice>Array of Double</Choice>\r\n<Choice>Array of Single</Choice>\r\n<Choice>Array of I64</Choice>\r\n<Choice>Array of I32</Choice>\r\n<Choice>Array of I16</Choice>\r\n<Choice>Array of I8</Choice>\r\n<Choice>Array of U64</Choice>\r\n<Choice>Array of U32</Choice>\r\n<Choice>Array of U16</Choice>\r\n<Choice>Array of U8</Choice>\r\n<Choice>Array of Boolean</Choice>\r\n<Choice>Array of String</Choice>\r\n<Val>0</Val>\r\n</EW>\r\n<Object>\r\n<Name>channel</Name>\r\n<NumLevels>2</NumLevels>\r\n<Class>TBM channel.lvclass</Class>\r\n<Version>1.0.0.3</Version>\r\n<Version>1.0.0.4</Version>\r\n<Cluster>\r\n<Name>tag descriptor.lvclass</Name>\r\n<NumElts>4</NumElts>\r\n<String>\r\n<Name>name</Name>\r\n<Val>AO8</Val>\r\n</String>\r\n<EW>\r\n<Name>data type</Name>\r\n<Choice>Double</Choice>\r\n<Choice>Single</Choice>\r\n<Choice>I64</Choice>\r\n<Choice>I32</Choice>\r\n<Choice>I16</Choice>\r\n<Choice>I8</Choice>\r\n<Choice>U64</Choice>\r\n<Choice>U32</Choice>\r\n<Choice>U16</Choice>\r\n<Choice>U8</Choice>\r\n<Choice>Boolean</Choice>\r\n<Choice>String</Choice>\r\n<Choice>Array of Double</Choice>\r\n<Choice>Array of Single</Choice>\r\n<Choice>Array of I64</Choice>\r\n<Choice>Array of I32</Choice>\r\n<Choice>Array of I16</Choice>\r\n<Choice>Array of I8</Choice>\r\n<Choice>Array of U64</Choice>\r\n<Choice>Array of U32</Choice>\r\n<Choice>Array of U16</Choice>\r\n<Choice>Array of U8</Choice>\r\n<Choice>Array of Boolean</Choice>\r\n<Choice>Array of String</Choice>\r\n<Val>0</Val>\r\n</EW>\r\n<String>\r\n<Name>default</Name>\r\n<Val></Val>\r\n</String>\r\n<String>\r\n<Name>metadata</Name>\r\n<Val></Val>\r\n</String>\r\n</Cluster>\r\n<Cluster>\r\n</Cluster>\r\n</Object>\r\n</Cluster>\r\n<Cluster>\r\n<Name>alarm config</Name>\r\n<NumElts>3</NumElts>\r\n<String>\r\n<Name>name</Name>\r\n<Val>AO9</Val>\r\n</String>\r\n<EW>\r\n<Name>data type</Name>\r\n<Choice>Double</Choice>\r\n<Choice>Single</Choice>\r\n<Choice>I64</Choice>\r\n<Choice>I32</Choice>\r\n<Choice>I16</Choice>\r\n<Choice>I8</Choice>\r\n<Choice>U64</Choice>\r\n<Choice>U32</Choice>\r\n<Choice>U16</Choice>\r\n<Choice>U8</Choice>\r\n<Choice>Boolean</Choice>\r\n<Choice>String</Choice>\r\n<Choice>Array of Double</Choice>\r\n<Choice>Array of Single</Choice>\r\n<Choice>Array of I64</Choice>\r\n<Choice>Array of I32</Choice>\r\n<Choice>Array of I16</Choice>\r\n<Choice>Array of I8</Choice>\r\n<Choice>Array of U64</Choice>\r\n<Choice>Array of U32</Choice>\r\n<Choice>Array of U16</Choice>\r\n<Choice>Array of U8</Choice>\r\n<Choice>Array of Boolean</Choice>\r\n<Choice>Array of String</Choice>\r\n<Val>10</Val>\r\n</EW>\r\n<Object>\r\n<Name>channel</Name>\r\n<NumLevels>2</NumLevels>\r\n<Class>TBM channel.lvclass</Class>\r\n<Version>1.0.0.3</Version>\r\n<Version>1.0.0.4</Version>\r\n<Cluster>\r\n<Name>tag descriptor.lvclass</Name>\r\n<NumElts>4</NumElts>\r\n<String>\r\n<Name>name</Name>\r\n<Val>AO9</Val>\r\n</String>\r\n<EW>\r\n<Name>data type</Name>\r\n<Choice>Double</Choice>\r\n<Choice>Single</Choice>\r\n<Choice>I64</Choice>\r\n<Choice>I32</Choice>\r\n<Choice>I16</Choice>\r\n<Choice>I8</Choice>\r\n<Choice>U64</Choice>\r\n<Choice>U32</Choice>\r\n<Choice>U16</Choice>\r\n<Choice>U8</Choice>\r\n<Choice>Boolean</Choice>\r\n<Choice>String</Choice>\r\n<Choice>Array of Double</Choice>\r\n<Choice>Array of Single</Choice>\r\n<Choice>Array of I64</Choice>\r\n<Choice>Array of I32</Choice>\r\n<Choice>Array of I16</Choice>\r\n<Choice>Array of I8</Choice>\r\n<Choice>Array of U64</Choice>\r\n<Choice>Array of U32</Choice>\r\n<Choice>Array of U16</Choice>\r\n<Choice>Array of U8</Choice>\r\n<Choice>Array of Boolean</Choice>\r\n<Choice>Array of String</Choice>\r\n<Val>10</Val>\r\n</EW>\r\n<String>\r\n<Name>default</Name>\r\n<Val></Val>\r\n</String>\r\n<String>\r\n<Name>metadata</Name>\r\n<Val></Val>\r\n</String>\r\n</Cluster>\r\n<Cluster>\r\n</Cluster>\r\n</Object>\r\n</Cluster>\r\n<Cluster>\r\n<Name>alarm config</Name>\r\n<NumElts>3</NumElts>\r\n<String>\r\n<Name>name</Name>\r\n<Val>AI10</Val>\r\n</String>\r\n<EW>\r\n<Name>data type</Name>\r\n<Choice>Double</Choice>\r\n<Choice>Single</Choice>\r\n<Choice>I64</Choice>\r\n<Choice>I32</Choice>\r\n<Choice>I16</Choice>\r\n<Choice>I8</Choice>\r\n<Choice>U64</Choice>\r\n<Choice>U32</Choice>\r\n<Choice>U16</Choice>\r\n<Choice>U8</Choice>\r\n<Choice>Boolean</Choice>\r\n<Choice>String</Choice>\r\n<Choice>Array of Double</Choice>\r\n<Choice>Array of Single</Choice>\r\n<Choice>Array of I64</Choice>\r\n<Choice>Array of I32</Choice>\r\n<Choice>Array of I16</Choice>\r\n<Choice>Array of I8</Choice>\r\n<Choice>Array of U64</Choice>\r\n<Choice>Array of U32</Choice>\r\n<Choice>Array of U16</Choice>\r\n<Choice>Array of U8</Choice>\r\n<Choice>Array of Boolean</Choice>\r\n<Choice>Array of String</Choice>\r\n<Val>3</Val>\r\n</EW>\r\n<Object>\r\n<Name>channel</Name>\r\n<NumLevels>2</NumLevels>\r\n<Class>TBM channel.lvclass</Class>\r\n<Version>1.0.0.3</Version>\r\n<Version>1.0.0.4</Version>\r\n<Cluster>\r\n<Name>tag descriptor.lvclass</Name>\r\n<NumElts>4</NumElts>\r\n<String>\r\n<Name>name</Name>\r\n<Val>AI10</Val>\r\n</String>\r\n<EW>\r\n<Name>data type</Name>\r\n<Choice>Double</Choice>\r\n<Choice>Single</Choice>\r\n<Choice>I64</Choice>\r\n<Choice>I32</Choice>\r\n<Choice>I16</Choice>\r\n<Choice>I8</Choice>\r\n<Choice>U64</Choice>\r\n<Choice>U32</Choice>\r\n<Choice>U16</Choice>\r\n<Choice>U8</Choice>\r\n<Choice>Boolean</Choice>\r\n<Choice>String</Choice>\r\n<Choice>Array of Double</Choice>\r\n<Choice>Array of Single</Choice>\r\n<Choice>Array of I64</Choice>\r\n<Choice>Array of I32</Choice>\r\n<Choice>Array of I16</Choice>\r\n<Choice>Array of I8</Choice>\r\n<Choice>Array of U64</Choice>\r\n<Choice>Array of U32</Choice>\r\n<Choice>Array of U16</Choice>\r\n<Choice>Array of U8</Choice>\r\n<Choice>Array of Boolean</Choice>\r\n<Choice>Array of String</Choice>\r\n<Val>3</Val>\r\n</EW>\r\n<String>\r\n<Name>default</Name>\r\n<Val></Val>\r\n</String>\r\n<String>\r\n<Name>metadata</Name>\r\n<Val></Val>\r\n</String>\r\n</Cluster>\r\n<Cluster>\r\n<Name>TBM channel.lvclass</Name>\r\n<NumElts>1</NumElts>\r\n<EW>\r\n<Name>channel classification</Name>\r\n<Choice>input data</Choice>\r\n<Choice>output data</Choice>\r\n<Choice>processing parameter</Choice>\r\n<Choice>processing result</Choice>\r\n<Val>1</Val>\r\n</EW>\r\n</Cluster>\r\n</Object>\r\n</Cluster>\r\n<Cluster>\r\n<Name>alarm config</Name>\r\n<NumElts>3</NumElts>\r\n<String>\r\n<Name>name</Name>\r\n<Val>AI11</Val>\r\n</String>\r\n<EW>\r\n<Name>data type</Name>\r\n<Choice>Double</Choice>\r\n<Choice>Single</Choice>\r\n<Choice>I64</Choice>\r\n<Choice>I32</Choice>\r\n<Choice>I16</Choice>\r\n<Choice>I8</Choice>\r\n<Choice>U64</Choice>\r\n<Choice>U32</Choice>\r\n<Choice>U16</Choice>\r\n<Choice>U8</Choice>\r\n<Choice>Boolean</Choice>\r\n<Choice>String</Choice>\r\n<Choice>Array of Double</Choice>\r\n<Choice>Array of Single</Choice>\r\n<Choice>Array of I64</Choice>\r\n<Choice>Array of I32</Choice>\r\n<Choice>Array of I16</Choice>\r\n<Choice>Array of I8</Choice>\r\n<Choice>Array of U64</Choice>\r\n<Choice>Array of U32</Choice>\r\n<Choice>Array of U16</Choice>\r\n<Choice>Array of U8</Choice>\r\n<Choice>Array of Boolean</Choice>\r\n<Choice>Array of String</Choice>\r\n<Val>0</Val>\r\n</EW>\r\n<Object>\r\n<Name>channel</Name>\r\n<NumLevels>2</NumLevels>\r\n<Class>TBM channel.lvclass</Class>\r\n<Version>1.0.0.3</Version>\r\n<Version>1.0.0.4</Version>\r\n<Cluster>\r\n<Name>tag descriptor.lvclass</Name>\r\n<NumElts>4</NumElts>\r\n<String>\r\n<Name>name</Name>\r\n<Val>AI11</Val>\r\n</String>\r\n<EW>\r\n<Name>data type</Name>\r\n<Choice>Double</Choice>\r\n<Choice>Single</Choice>\r\n<Choice>I64</Choice>\r\n<Choice>I32</Choice>\r\n<Choice>I16</Choice>\r\n<Choice>I8</Choice>\r\n<Choice>U64</Choice>\r\n<Choice>U32</Choice>\r\n<Choice>U16</Choice>\r\n<Choice>U8</Choice>\r\n<Choice>Boolean</Choice>\r\n<Choice>String</Choice>\r\n<Choice>Array of Double</Choice>\r\n<Choice>Array of Single</Choice>\r\n<Choice>Array of I64</Choice>\r\n<Choice>Array of I32</Choice>\r\n<Choice>Array of I16</Choice>\r\n<Choice>Array of I8</Choice>\r\n<Choice>Array of U64</Choice>\r\n<Choice>Array of U32</Choice>\r\n<Choice>Array of U16</Choice>\r\n<Choice>Array of U8</Choice>\r\n<Choice>Array of Boolean</Choice>\r\n<Choice>Array of String</Choice>\r\n<Val>0</Val>\r\n</EW>\r\n<String>\r\n<Name>default</Name>\r\n<Val></Val>\r\n</String>\r\n<String>\r\n<Name>metadata</Name>\r\n<Val></Val>\r\n</String>\r\n</Cluster>\r\n<Cluster>\r\n<Name>TBM channel.lvclass</Name>\r\n<NumElts>1</NumElts>\r\n<EW>\r\n<Name>channel classification</Name>\r\n<Choice>input data</Choice>\r\n<Choice>output data</Choice>\r\n<Choice>processing parameter</Choice>\r\n<Choice>processing result</Choice>\r\n<Val>1</Val>\r\n</EW>\r\n</Cluster>\r\n</Object>\r\n</Cluster>\r\n<Cluster>\r\n<Name>alarm config</Name>\r\n<NumElts>3</NumElts>\r\n<String>\r\n<Name>name</Name>\r\n<Val>AI12</Val>\r\n</String>\r\n<EW>\r\n<Name>data type</Name>\r\n<Choice>Double</Choice>\r\n<Choice>Single</Choice>\r\n<Choice>I64</Choice>\r\n<Choice>I32</Choice>\r\n<Choice>I16</Choice>\r\n<Choice>I8</Choice>\r\n<Choice>U64</Choice>\r\n<Choice>U32</Choice>\r\n<Choice>U16</Choice>\r\n<Choice>U8</Choice>\r\n<Choice>Boolean</Choice>\r\n<Choice>String</Choice>\r\n<Choice>Array of Double</Choice>\r\n<Choice>Array of Single</Choice>\r\n<Choice>Array of I64</Choice>\r\n<Choice>Array of I32</Choice>\r\n<Choice>Array of I16</Choice>\r\n<Choice>Array of I8</Choice>\r\n<Choice>Array of U64</Choice>\r\n<Choice>Array of U32</Choice>\r\n<Choice>Array of U16</Choice>\r\n<Choice>Array of U8</Choice>\r\n<Choice>Array of Boolean</Choice>\r\n<Choice>Array of String</Choice>\r\n<Val>10</Val>\r\n</EW>\r\n<Object>\r\n<Name>channel</Name>\r\n<NumLevels>2</NumLevels>\r\n<Class>TBM channel.lvclass</Class>\r\n<Version>1.0.0.3</Version>\r\n<Version>1.0.0.4</Version>\r\n<Cluster>\r\n<Name>tag descriptor.lvclass</Name>\r\n<NumElts>4</NumElts>\r\n<String>\r\n<Name>name</Name>\r\n<Val>AI12</Val>\r\n</String>\r\n<EW>\r\n<Name>data type</Name>\r\n<Choice>Double</Choice>\r\n<Choice>Single</Choice>\r\n<Choice>I64</Choice>\r\n<Choice>I32</Choice>\r\n<Choice>I16</Choice>\r\n<Choice>I8</Choice>\r\n<Choice>U64</Choice>\r\n<Choice>U32</Choice>\r\n<Choice>U16</Choice>\r\n<Choice>U8</Choice>\r\n<Choice>Boolean</Choice>\r\n<Choice>String</Choice>\r\n<Choice>Array of Double</Choice>\r\n<Choice>Array of Single</Choice>\r\n<Choice>Array of I64</Choice>\r\n<Choice>Array of I32</Choice>\r\n<Choice>Array of I16</Choice>\r\n<Choice>Array of I8</Choice>\r\n<Choice>Array of U64</Choice>\r\n<Choice>Array of U32</Choice>\r\n<Choice>Array of U16</Choice>\r\n<Choice>Array of U8</Choice>\r\n<Choice>Array of Boolean</Choice>\r\n<Choice>Array of String</Choice>\r\n<Val>10</Val>\r\n</EW>\r\n<String>\r\n<Name>default</Name>\r\n<Val></Val>\r\n</String>\r\n<String>\r\n<Name>metadata</Name>\r\n<Val></Val>\r\n</String>\r\n</Cluster>\r\n<Cluster>\r\n<Name>TBM channel.lvclass</Name>\r\n<NumElts>1</NumElts>\r\n<EW>\r\n<Name>channel classification</Name>\r\n<Choice>input data</Choice>\r\n<Choice>output data</Choice>\r\n<Choice>processing parameter</Choice>\r\n<Choice>processing result</Choice>\r\n<Val>1</Val>\r\n</EW>\r\n</Cluster>\r\n</Object>\r\n</Cluster>\r\n<Cluster>\r\n<Name>alarm config</Name>\r\n<NumElts>3</NumElts>\r\n<String>\r\n<Name>name</Name>\r\n<Val>AI13</Val>\r\n</String>\r\n<EW>\r\n<Name>data type</Name>\r\n<Choice>Double</Choice>\r\n<Choice>Single</Choice>\r\n<Choice>I64</Choice>\r\n<Choice>I32</Choice>\r\n<Choice>I16</Choice>\r\n<Choice>I8</Choice>\r\n<Choice>U64</Choice>\r\n<Choice>U32</Choice>\r\n<Choice>U16</Choice>\r\n<Choice>U8</Choice>\r\n<Choice>Boolean</Choice>\r\n<Choice>String</Choice>\r\n<Choice>Array of Double</Choice>\r\n<Choice>Array of Single</Choice>\r\n<Choice>Array of I64</Choice>\r\n<Choice>Array of I32</Choice>\r\n<Choice>Array of I16</Choice>\r\n<Choice>Array of I8</Choice>\r\n<Choice>Array of U64</Choice>\r\n<Choice>Array of U32</Choice>\r\n<Choice>Array of U16</Choice>\r\n<Choice>Array of U8</Choice>\r\n<Choice>Array of Boolean</Choice>\r\n<Choice>Array of String</Choice>\r\n<Val>3</Val>\r\n</EW>\r\n<Object>\r\n<Name>channel</Name>\r\n<NumLevels>2</NumLevels>\r\n<Class>TBM channel.lvclass</Class>\r\n<Version>1.0.0.3</Version>\r\n<Version>1.0.0.4</Version>\r\n<Cluster>\r\n<Name>tag descriptor.lvclass</Name>\r\n<NumElts>4</NumElts>\r\n<String>\r\n<Name>name</Name>\r\n<Val>AI13</Val>\r\n</String>\r\n<EW>\r\n<Name>data type</Name>\r\n<Choice>Double</Choice>\r\n<Choice>Single</Choice>\r\n<Choice>I64</Choice>\r\n<Choice>I32</Choice>\r\n<Choice>I16</Choice>\r\n<Choice>I8</Choice>\r\n<Choice>U64</Choice>\r\n<Choice>U32</Choice>\r\n<Choice>U16</Choice>\r\n<Choice>U8</Choice>\r\n<Choice>Boolean</Choice>\r\n<Choice>String</Choice>\r\n<Choice>Array of Double</Choice>\r\n<Choice>Array of Single</Choice>\r\n<Choice>Array of I64</Choice>\r\n<Choice>Array of I32</Choice>\r\n<Choice>Array of I16</Choice>\r\n<Choice>Array of I8</Choice>\r\n<Choice>Array of U64</Choice>\r\n<Choice>Array of U32</Choice>\r\n<Choice>Array of U16</Choice>\r\n<Choice>Array of U8</Choice>\r\n<Choice>Array of Boolean</Choice>\r\n<Choice>Array of String</Choice>\r\n<Val>3</Val>\r\n</EW>\r\n<String>\r\n<Name>default</Name>\r\n<Val></Val>\r\n</String>\r\n<String>\r\n<Name>metadata</Name>\r\n<Val></Val>\r\n</String>\r\n</Cluster>\r\n<Cluster>\r\n<Name>TBM channel.lvclass</Name>\r\n<NumElts>1</NumElts>\r\n<EW>\r\n<Name>channel classification</Name>\r\n<Choice>input data</Choice>\r\n<Choice>output data</Choice>\r\n<Choice>processing parameter</Choice>\r\n<Choice>processing result</Choice>\r\n<Val>1</Val>\r\n</EW>\r\n</Cluster>\r\n</Object>\r\n</Cluster>\r\n<Cluster>\r\n<Name>alarm config</Name>\r\n<NumElts>3</NumElts>\r\n<String>\r\n<Name>name</Name>\r\n<Val>AI14</Val>\r\n</String>\r\n<EW>\r\n<Name>data type</Name>\r\n<Choice>Double</Choice>\r\n<Choice>Single</Choice>\r\n<Choice>I64</Choice>\r\n<Choice>I32</Choice>\r\n<Choice>I16</Choice>\r\n<Choice>I8</Choice>\r\n<Choice>U64</Choice>\r\n<Choice>U32</Choice>\r\n<Choice>U16</Choice>\r\n<Choice>U8</Choice>\r\n<Choice>Boolean</Choice>\r\n<Choice>String</Choice>\r\n<Choice>Array of Double</Choice>\r\n<Choice>Array of Single</Choice>\r\n<Choice>Array of I64</Choice>\r\n<Choice>Array of I32</Choice>\r\n<Choice>Array of I16</Choice>\r\n<Choice>Array of I8</Choice>\r\n<Choice>Array of U64</Choice>\r\n<Choice>Array of U32</Choice>\r\n<Choice>Array of U16</Choice>\r\n<Choice>Array of U8</Choice>\r\n<Choice>Array of Boolean</Choice>\r\n<Choice>Array of String</Choice>\r\n<Val>0</Val>\r\n</EW>\r\n<Object>\r\n<Name>channel</Name>\r\n<NumLevels>2</NumLevels>\r\n<Class>TBM channel.lvclass</Class>\r\n<Version>1.0.0.3</Version>\r\n<Version>1.0.0.4</Version>\r\n<Cluster>\r\n<Name>tag descriptor.lvclass</Name>\r\n<NumElts>4</NumElts>\r\n<String>\r\n<Name>name</Name>\r\n<Val>AI14</Val>\r\n</String>\r\n<EW>\r\n<Name>data type</Name>\r\n<Choice>Double</Choice>\r\n<Choice>Single</Choice>\r\n<Choice>I64</Choice>\r\n<Choice>I32</Choice>\r\n<Choice>I16</Choice>\r\n<Choice>I8</Choice>\r\n<Choice>U64</Choice>\r\n<Choice>U32</Choice>\r\n<Choice>U16</Choice>\r\n<Choice>U8</Choice>\r\n<Choice>Boolean</Choice>\r\n<Choice>String</Choice>\r\n<Choice>Array of Double</Choice>\r\n<Choice>Array of Single</Choice>\r\n<Choice>Array of I64</Choice>\r\n<Choice>Array of I32</Choice>\r\n<Choice>Array of I16</Choice>\r\n<Choice>Array of I8</Choice>\r\n<Choice>Array of U64</Choice>\r\n<Choice>Array of U32</Choice>\r\n<Choice>Array of U16</Choice>\r\n<Choice>Array of U8</Choice>\r\n<Choice>Array of Boolean</Choice>\r\n<Choice>Array of String</Choice>\r\n<Val>0</Val>\r\n</EW>\r\n<String>\r\n<Name>default</Name>\r\n<Val></Val>\r\n</String>\r\n<String>\r\n<Name>metadata</Name>\r\n<Val></Val>\r\n</String>\r\n</Cluster>\r\n<Cluster>\r\n<Name>TBM channel.lvclass</Name>\r\n<NumElts>1</NumElts>\r\n<EW>\r\n<Name>channel classification</Name>\r\n<Choice>input data</Choice>\r\n<Choice>output data</Choice>\r\n<Choice>processing parameter</Choice>\r\n<Choice>processing result</Choice>\r\n<Val>1</Val>\r\n</EW>\r\n</Cluster>\r\n</Object>\r\n</Cluster>\r\n<Cluster>\r\n<Name>alarm config</Name>\r\n<NumElts>3</NumElts>\r\n<String>\r\n<Name>name</Name>\r\n<Val>AI15</Val>\r\n</String>\r\n<EW>\r\n<Name>data type</Name>\r\n<Choice>Double</Choice>\r\n<Choice>Single</Choice>\r\n<Choice>I64</Choice>\r\n<Choice>I32</Choice>\r\n<Choice>I16</Choice>\r\n<Choice>I8</Choice>\r\n<Choice>U64</Choice>\r\n<Choice>U32</Choice>\r\n<Choice>U16</Choice>\r\n<Choice>U8</Choice>\r\n<Choice>Boolean</Choice>\r\n<Choice>String</Choice>\r\n<Choice>Array of Double</Choice>\r\n<Choice>Array of Single</Choice>\r\n<Choice>Array of I64</Choice>\r\n<Choice>Array of I32</Choice>\r\n<Choice>Array of I16</Choice>\r\n<Choice>Array of I8</Choice>\r\n<Choice>Array of U64</Choice>\r\n<Choice>Array of U32</Choice>\r\n<Choice>Array of U16</Choice>\r\n<Choice>Array of U8</Choice>\r\n<Choice>Array of Boolean</Choice>\r\n<Choice>Array of String</Choice>\r\n<Val>10</Val>\r\n</EW>\r\n<Object>\r\n<Name>channel</Name>\r\n<NumLevels>2</NumLevels>\r\n<Class>TBM channel.lvclass</Class>\r\n<Version>1.0.0.3</Version>\r\n<Version>1.0.0.4</Version>\r\n<Cluster>\r\n<Name>tag descriptor.lvclass</Name>\r\n<NumElts>4</NumElts>\r\n<String>\r\n<Name>name</Name>\r\n<Val>AI15</Val>\r\n</String>\r\n<EW>\r\n<Name>data type</Name>\r\n<Choice>Double</Choice>\r\n<Choice>Single</Choice>\r\n<Choice>I64</Choice>\r\n<Choice>I32</Choice>\r\n<Choice>I16</Choice>\r\n<Choice>I8</Choice>\r\n<Choice>U64</Choice>\r\n<Choice>U32</Choice>\r\n<Choice>U16</Choice>\r\n<Choice>U8</Choice>\r\n<Choice>Boolean</Choice>\r\n<Choice>String</Choice>\r\n<Choice>Array of Double</Choice>\r\n<Choice>Array of Single</Choice>\r\n<Choice>Array of I64</Choice>\r\n<Choice>Array of I32</Choice>\r\n<Choice>Array of I16</Choice>\r\n<Choice>Array of I8</Choice>\r\n<Choice>Array of U64</Choice>\r\n<Choice>Array of U32</Choice>\r\n<Choice>Array of U16</Choice>\r\n<Choice>Array of U8</Choice>\r\n<Choice>Array of Boolean</Choice>\r\n<Choice>Array of String</Choice>\r\n<Val>10</Val>\r\n</EW>\r\n<String>\r\n<Name>default</Name>\r\n<Val></Val>\r\n</String>\r\n<String>\r\n<Name>metadata</Name>\r\n<Val></Val>\r\n</String>\r\n</Cluster>\r\n<Cluster>\r\n<Name>TBM channel.lvclass</Name>\r\n<NumElts>1</NumElts>\r\n<EW>\r\n<Name>channel classification</Name>\r\n<Choice>input data</Choice>\r\n<Choice>output data</Choice>\r\n<Choice>processing parameter</Choice>\r\n<Choice>processing result</Choice>\r\n<Val>1</Val>\r\n</EW>\r\n</Cluster>\r\n</Object>\r\n</Cluster>\r\n<Cluster>\r\n<Name>alarm config</Name>\r\n<NumElts>3</NumElts>\r\n<String>\r\n<Name>name</Name>\r\n<Val>AI16</Val>\r\n</String>\r\n<EW>\r\n<Name>data type</Name>\r\n<Choice>Double</Choice>\r\n<Choice>Single</Choice>\r\n<Choice>I64</Choice>\r\n<Choice>I32</Choice>\r\n<Choice>I16</Choice>\r\n<Choice>I8</Choice>\r\n<Choice>U64</Choice>\r\n<Choice>U32</Choice>\r\n<Choice>U16</Choice>\r\n<Choice>U8</Choice>\r\n<Choice>Boolean</Choice>\r\n<Choice>String</Choice>\r\n<Choice>Array of Double</Choice>\r\n<Choice>Array of Single</Choice>\r\n<Choice>Array of I64</Choice>\r\n<Choice>Array of I32</Choice>\r\n<Choice>Array of I16</Choice>\r\n<Choice>Array of I8</Choice>\r\n<Choice>Array of U64</Choice>\r\n<Choice>Array of U32</Choice>\r\n<Choice>Array of U16</Choice>\r\n<Choice>Array of U8</Choice>\r\n<Choice>Array of Boolean</Choice>\r\n<Choice>Array of String</Choice>\r\n<Val>3</Val>\r\n</EW>\r\n<Object>\r\n<Name>channel</Name>\r\n<NumLevels>2</NumLevels>\r\n<Class>TBM channel.lvclass</Class>\r\n<Version>1.0.0.3</Version>\r\n<Version>1.0.0.4</Version>\r\n<Cluster>\r\n<Name>tag descriptor.lvclass</Name>\r\n<NumElts>4</NumElts>\r\n<String>\r\n<Name>name</Name>\r\n<Val>AI16</Val>\r\n</String>\r\n<EW>\r\n<Name>data type</Name>\r\n<Choice>Double</Choice>\r\n<Choice>Single</Choice>\r\n<Choice>I64</Choice>\r\n<Choice>I32</Choice>\r\n<Choice>I16</Choice>\r\n<Choice>I8</Choice>\r\n<Choice>U64</Choice>\r\n<Choice>U32</Choice>\r\n<Choice>U16</Choice>\r\n<Choice>U8</Choice>\r\n<Choice>Boolean</Choice>\r\n<Choice>String</Choice>\r\n<Choice>Array of Double</Choice>\r\n<Choice>Array of Single</Choice>\r\n<Choice>Array of I64</Choice>\r\n<Choice>Array of I32</Choice>\r\n<Choice>Array of I16</Choice>\r\n<Choice>Array of I8</Choice>\r\n<Choice>Array of U64</Choice>\r\n<Choice>Array of U32</Choice>\r\n<Choice>Array of U16</Choice>\r\n<Choice>Array of U8</Choice>\r\n<Choice>Array of Boolean</Choice>\r\n<Choice>Array of String</Choice>\r\n<Val>3</Val>\r\n</EW>\r\n<String>\r\n<Name>default</Name>\r\n<Val></Val>\r\n</String>\r\n<String>\r\n<Name>metadata</Name>\r\n<Val></Val>\r\n</String>\r\n</Cluster>\r\n<Cluster>\r\n<Name>TBM channel.lvclass</Name>\r\n<NumElts>1</NumElts>\r\n<EW>\r\n<Name>channel classification</Name>\r\n<Choice>input data</Choice>\r\n<Choice>output data</Choice>\r\n<Choice>processing parameter</Choice>\r\n<Choice>processing result</Choice>\r\n<Val>1</Val>\r\n</EW>\r\n</Cluster>\r\n</Object>\r\n</Cluster>\r\n<Cluster>\r\n<Name>alarm config</Name>\r\n<NumElts>3</NumElts>\r\n<String>\r\n<Name>name</Name>\r\n<Val>AI17</Val>\r\n</String>\r\n<EW>\r\n<Name>data type</Name>\r\n<Choice>Double</Choice>\r\n<Choice>Single</Choice>\r\n<Choice>I64</Choice>\r\n<Choice>I32</Choice>\r\n<Choice>I16</Choice>\r\n<Choice>I8</Choice>\r\n<Choice>U64</Choice>\r\n<Choice>U32</Choice>\r\n<Choice>U16</Choice>\r\n<Choice>U8</Choice>\r\n<Choice>Boolean</Choice>\r\n<Choice>String</Choice>\r\n<Choice>Array of Double</Choice>\r\n<Choice>Array of Single</Choice>\r\n<Choice>Array of I64</Choice>\r\n<Choice>Array of I32</Choice>\r\n<Choice>Array of I16</Choice>\r\n<Choice>Array of I8</Choice>\r\n<Choice>Array of U64</Choice>\r\n<Choice>Array of U32</Choice>\r\n<Choice>Array of U16</Choice>\r\n<Choice>Array of U8</Choice>\r\n<Choice>Array of Boolean</Choice>\r\n<Choice>Array of String</Choice>\r\n<Val>0</Val>\r\n</EW>\r\n<Object>\r\n<Name>channel</Name>\r\n<NumLevels>2</NumLevels>\r\n<Class>TBM channel.lvclass</Class>\r\n<Version>1.0.0.3</Version>\r\n<Version>1.0.0.4</Version>\r\n<Cluster>\r\n<Name>tag descriptor.lvclass</Name>\r\n<NumElts>4</NumElts>\r\n<String>\r\n<Name>name</Name>\r\n<Val>AI17</Val>\r\n</String>\r\n<EW>\r\n<Name>data type</Name>\r\n<Choice>Double</Choice>\r\n<Choice>Single</Choice>\r\n<Choice>I64</Choice>\r\n<Choice>I32</Choice>\r\n<Choice>I16</Choice>\r\n<Choice>I8</Choice>\r\n<Choice>U64</Choice>\r\n<Choice>U32</Choice>\r\n<Choice>U16</Choice>\r\n<Choice>U8</Choice>\r\n<Choice>Boolean</Choice>\r\n<Choice>String</Choice>\r\n<Choice>Array of Double</Choice>\r\n<Choice>Array of Single</Choice>\r\n<Choice>Array of I64</Choice>\r\n<Choice>Array of I32</Choice>\r\n<Choice>Array of I16</Choice>\r\n<Choice>Array of I8</Choice>\r\n<Choice>Array of U64</Choice>\r\n<Choice>Array of U32</Choice>\r\n<Choice>Array of U16</Choice>\r\n<Choice>Array of U8</Choice>\r\n<Choice>Array of Boolean</Choice>\r\n<Choice>Array of String</Choice>\r\n<Val>0</Val>\r\n</EW>\r\n<String>\r\n<Name>default</Name>\r\n<Val></Val>\r\n</String>\r\n<String>\r\n<Name>metadata</Name>\r\n<Val></Val>\r\n</String>\r\n</Cluster>\r\n<Cluster>\r\n<Name>TBM channel.lvclass</Name>\r\n<NumElts>1</NumElts>\r\n<EW>\r\n<Name>channel classification</Name>\r\n<Choice>input data</Choice>\r\n<Choice>output data</Choice>\r\n<Choice>processing parameter</Choice>\r\n<Choice>processing result</Choice>\r\n<Val>1</Val>\r\n</EW>\r\n</Cluster>\r\n</Object>\r\n</Cluster>\r\n<Cluster>\r\n<Name>alarm config</Name>\r\n<NumElts>3</NumElts>\r\n<String>\r\n<Name>name</Name>\r\n<Val>AI18</Val>\r\n</String>\r\n<EW>\r\n<Name>data type</Name>\r\n<Choice>Double</Choice>\r\n<Choice>Single</Choice>\r\n<Choice>I64</Choice>\r\n<Choice>I32</Choice>\r\n<Choice>I16</Choice>\r\n<Choice>I8</Choice>\r\n<Choice>U64</Choice>\r\n<Choice>U32</Choice>\r\n<Choice>U16</Choice>\r\n<Choice>U8</Choice>\r\n<Choice>Boolean</Choice>\r\n<Choice>String</Choice>\r\n<Choice>Array of Double</Choice>\r\n<Choice>Array of Single</Choice>\r\n<Choice>Array of I64</Choice>\r\n<Choice>Array of I32</Choice>\r\n<Choice>Array of I16</Choice>\r\n<Choice>Array of I8</Choice>\r\n<Choice>Array of U64</Choice>\r\n<Choice>Array of U32</Choice>\r\n<Choice>Array of U16</Choice>\r\n<Choice>Array of U8</Choice>\r\n<Choice>Array of Boolean</Choice>\r\n<Choice>Array of String</Choice>\r\n<Val>10</Val>\r\n</EW>\r\n<Object>\r\n<Name>channel</Name>\r\n<NumLevels>2</NumLevels>\r\n<Class>TBM channel.lvclass</Class>\r\n<Version>1.0.0.3</Version>\r\n<Version>1.0.0.4</Version>\r\n<Cluster>\r\n<Name>tag descriptor.lvclass</Name>\r\n<NumElts>4</NumElts>\r\n<String>\r\n<Name>name</Name>\r\n<Val>AI18</Val>\r\n</String>\r\n<EW>\r\n<Name>data type</Name>\r\n<Choice>Double</Choice>\r\n<Choice>Single</Choice>\r\n<Choice>I64</Choice>\r\n<Choice>I32</Choice>\r\n<Choice>I16</Choice>\r\n<Choice>I8</Choice>\r\n<Choice>U64</Choice>\r\n<Choice>U32</Choice>\r\n<Choice>U16</Choice>\r\n<Choice>U8</Choice>\r\n<Choice>Boolean</Choice>\r\n<Choice>String</Choice>\r\n<Choice>Array of Double</Choice>\r\n<Choice>Array of Single</Choice>\r\n<Choice>Array of I64</Choice>\r\n<Choice>Array of I32</Choice>\r\n<Choice>Array of I16</Choice>\r\n<Choice>Array of I8</Choice>\r\n<Choice>Array of U64</Choice>\r\n<Choice>Array of U32</Choice>\r\n<Choice>Array of U16</Choice>\r\n<Choice>Array of U8</Choice>\r\n<Choice>Array of Boolean</Choice>\r\n<Choice>Array of String</Choice>\r\n<Val>10</Val>\r\n</EW>\r\n<String>\r\n<Name>default</Name>\r\n<Val></Val>\r\n</String>\r\n<String>\r\n<Name>metadata</Name>\r\n<Val></Val>\r\n</String>\r\n</Cluster>\r\n<Cluster>\r\n<Name>TBM channel.lvclass</Name>\r\n<NumElts>1</NumElts>\r\n<EW>\r\n<Name>channel classification</Name>\r\n<Choice>input data</Choice>\r\n<Choice>output data</Choice>\r\n<Choice>processing parameter</Choice>\r\n<Choice>processing result</Choice>\r\n<Val>1</Val>\r\n</EW>\r\n</Cluster>\r\n</Object>\r\n</Cluster>\r\n<Cluster>\r\n<Name>alarm config</Name>\r\n<NumElts>3</NumElts>\r\n<String>\r\n<Name>name</Name>\r\n<Val>AI19</Val>\r\n</String>\r\n<EW>\r\n<Name>data type</Name>\r\n<Choice>Double</Choice>\r\n<Choice>Single</Choice>\r\n<Choice>I64</Choice>\r\n<Choice>I32</Choice>\r\n<Choice>I16</Choice>\r\n<Choice>I8</Choice>\r\n<Choice>U64</Choice>\r\n<Choice>U32</Choice>\r\n<Choice>U16</Choice>\r\n<Choice>U8</Choice>\r\n<Choice>Boolean</Choice>\r\n<Choice>String</Choice>\r\n<Choice>Array of Double</Choice>\r\n<Choice>Array of Single</Choice>\r\n<Choice>Array of I64</Choice>\r\n<Choice>Array of I32</Choice>\r\n<Choice>Array of I16</Choice>\r\n<Choice>Array of I8</Choice>\r\n<Choice>Array of U64</Choice>\r\n<Choice>Array of U32</Choice>\r\n<Choice>Array of U16</Choice>\r\n<Choice>Array of U8</Choice>\r\n<Choice>Array of Boolean</Choice>\r\n<Choice>Array of String</Choice>\r\n<Val>3</Val>\r\n</EW>\r\n<Object>\r\n<Name>channel</Name>\r\n<NumLevels>2</NumLevels>\r\n<Class>TBM channel.lvclass</Class>\r\n<Version>1.0.0.3</Version>\r\n<Version>1.0.0.4</Version>\r\n<Cluster>\r\n<Name>tag descriptor.lvclass</Name>\r\n<NumElts>4</NumElts>\r\n<String>\r\n<Name>name</Name>\r\n<Val>AI19</Val>\r\n</String>\r\n<EW>\r\n<Name>data type</Name>\r\n<Choice>Double</Choice>\r\n<Choice>Single</Choice>\r\n<Choice>I64</Choice>\r\n<Choice>I32</Choice>\r\n<Choice>I16</Choice>\r\n<Choice>I8</Choice>\r\n<Choice>U64</Choice>\r\n<Choice>U32</Choice>\r\n<Choice>U16</Choice>\r\n<Choice>U8</Choice>\r\n<Choice>Boolean</Choice>\r\n<Choice>String</Choice>\r\n<Choice>Array of Double</Choice>\r\n<Choice>Array of Single</Choice>\r\n<Choice>Array of I64</Choice>\r\n<Choice>Array of I32</Choice>\r\n<Choice>Array of I16</Choice>\r\n<Choice>Array of I8</Choice>\r\n<Choice>Array of U64</Choice>\r\n<Choice>Array of U32</Choice>\r\n<Choice>Array of U16</Choice>\r\n<Choice>Array of U8</Choice>\r\n<Choice>Array of Boolean</Choice>\r\n<Choice>Array of String</Choice>\r\n<Val>3</Val>\r\n</EW>\r\n<String>\r\n<Name>default</Name>\r\n<Val></Val>\r\n</String>\r\n<String>\r\n<Name>metadata</Name>\r\n<Val></Val>\r\n</String>\r\n</Cluster>\r\n<Cluster>\r\n<Name>TBM channel.lvclass</Name>\r\n<NumElts>1</NumElts>\r\n<EW>\r\n<Name>channel classification</Name>\r\n<Choice>input data</Choice>\r\n<Choice>output data</Choice>\r\n<Choice>processing parameter</Choice>\r\n<Choice>processing result</Choice>\r\n<Val>1</Val>\r\n</EW>\r\n</Cluster>\r\n</Object>\r\n</Cluster>\r\n</Array>\r\n<Path>\r\n<Name>read directory</Name>\r\n<Val>C:\\Users\\Lee\\Documents\\LabVIEW Data\\Engine\\output</Val>\r\n</Path>\r\n<Path>\r\n<Name>write directory</Name>\r\n<Val>C:\\Users\\Lee\\Documents\\LabVIEW Data\\Engine\\input</Val>\r\n</Path>\r\n</Cluster>\r\n</Shared Memory>", "version"="1.0.0.0") -> ("shared memory module configuration out"=w1:refnum<class "Shared Memory Configuration.lvclass">)  [unwired: 8 in, 1 out]
  n2 = call "channel add.vi"() -> ("error out"=w18:errorcluster)  [unwired: 7 in, 4 out]
  n3 = call-dynamic "init.vi"("error in"=w18, "TBM module configuration in"=w1, "shared memory module runtime"=refnum<class "Shared Memory Runtime.lvclass"> refnum ("tag bus configurable plugin module")) -> ("error out"=w17:errorcluster, "data allocations"=w12:T1, "shared memory module runtime out"=w16:refnum<class "Shared Memory Runtime.lvclass">)  [unwired: 5 in, 1 out]
  n4 = property class="Shared Memory Runtime"(reference=w16, error in=w17) -> (reference out=w7:refnum<class "Shared Memory Runtime.lvclass">, error out=w6:errorcluster, "Properties:inputs"=w9:T4[], "Properties:outputs"=w15:T4[])
  n5 = Unbundle By Name(w12) -> ("input data.data table"=w8:T3)
  n6 = for {
    shift-right: [w22] -> w5
    shift-left: w7 -> [w22]
    shift-right: [w21] -> w4
    shift-left: w6 -> [w21]
    shift-right: [w20] -> _
    shift-left: w8 -> [w28]
    tunnel: w9 -> [w26] mode=indexing
    n7 = Unbundle By Name(w26) -> ("data type"=w24:T5, "indices"=w25:cluster{"index":i32[]})
    n8 = Wait Until Next ms Multiple(millisecond multiple=u32 100) -> ()  [unwired: 1 out]
    n9 = Unbundle(w25) -> ("index"=w23:i32[])
    n10 = case shown="\"I64\"" w24 {
      tunnel: w28 -> [w34 w40 w46 w52 w58 w64 w70 w76 w82 w88 w94 w100 w101]
      tunnel: [w29 w35 w41 w47 w53 w59 w65 w71 w77 w83 w89 w95 w101] -> w20
      tunnel: w23 -> [w33 w39 w45 w51 w57 w63 w69 w75 w81 w87 w93 w99 _]
      frame "Double" {
        n11 = Array Size(array=w33) -> (size(s)=w32:i32)
        n12 = Initialize Array(0.0 ("element"), w32) -> (w30:dbl[])
        n13 = call-poly <vilib>:"write multiple elements.vi"("values"=w30, "indices"=w33, "data table in"=w34) -> ("data table out"=w29:T3)  [unwired: 8 in]
      }
      frame "Single" {
        n14 = Array Size(array=w39) -> (size(s)=w38:i32)
        n15 = Initialize Array(sgl 0.0 ("element"), w38) -> (w36:sgl[])
        n16 = call-poly <vilib>:"write multiple elements.vi"("values"=w36, "indices"=w39, "data table in"=w40) -> ("data table out"=w35:T3)  [unwired: 8 in]
      }
      frame "I64" {
        n17 = Array Size(array=w45) -> (size(s)=w44:i32)
        n18 = Initialize Array(i64 0 ("element"), w44) -> (w42:i64[])
        n19 = call-poly <vilib>:"write multiple elements.vi"("values"=w42, "indices"=w45, "data table in"=w46) -> ("data table out"=w41:T3)  [unwired: 8 in]
      }
      frame "I32" {
        n20 = Array Size(array=w51) -> (size(s)=w50:i32)
        n21 = Initialize Array(0 ("element"), w50) -> (w48:i32[])
        n22 = call-poly <vilib>:"write multiple elements.vi"("values"=w48, "indices"=w51, "data table in"=w52) -> ("data table out"=w47:T3)  [unwired: 8 in]
      }
      frame "I16" {
        n23 = Array Size(array=w57) -> (size(s)=w56:i32)
        n24 = Initialize Array(i16 0 ("element"), w56) -> (w54:i16[])
        n25 = call-poly <vilib>:"write multiple elements.vi"("values"=w54, "indices"=w57, "data table in"=w58) -> ("data table out"=w53:T3)  [unwired: 8 in]
      }
      frame "I8" {
        n26 = Array Size(array=w63) -> (size(s)=w62:i32)
        n27 = Initialize Array(i8 0 ("element"), w62) -> (w60:i8[])
        n28 = call-poly <vilib>:"write multiple elements.vi"("values"=w60, "indices"=w63, "data table in"=w64) -> ("data table out"=w59:T3)  [unwired: 8 in]
      }
      frame "U64" {
        n29 = Array Size(array=w69) -> (size(s)=w68:i32)
        n30 = Initialize Array(u64 0 ("element"), w68) -> (w66:u64[])
        n31 = call-poly <vilib>:"write multiple elements.vi"("values"=w66, "indices"=w69, "data table in"=w70) -> ("data table out"=w65:T3)  [unwired: 8 in]
      }
      frame "U32" {
        n32 = Array Size(array=w75) -> (size(s)=w74:i32)
        n33 = Initialize Array(u32 0 ("element"), w74) -> (w72:u32[])
        n34 = call-poly <vilib>:"write multiple elements.vi"("values"=w72, "indices"=w75, "data table in"=w76) -> ("data table out"=w71:T3)  [unwired: 8 in]
      }
      frame "U16" {
        n35 = Array Size(array=w81) -> (size(s)=w80:i32)
        n36 = Initialize Array(u16 0 ("element"), w80) -> (w78:u16[])
        n37 = call-poly <vilib>:"write multiple elements.vi"("values"=w78, "indices"=w81, "data table in"=w82) -> ("data table out"=w77:T3)  [unwired: 8 in]
      }
      frame "U8" {
        n38 = Array Size(array=w87) -> (size(s)=w86:i32)
        n39 = Initialize Array(u8 0 ("element"), w86) -> (w84:u8[])
        n40 = call-poly <vilib>:"write multiple elements.vi"("values"=w84, "indices"=w87, "data table in"=w88) -> ("data table out"=w83:T3)  [unwired: 8 in]
      }
      frame "String" {
        n41 = Array Size(array=w93) -> (size(s)=w92:i32)
        n42 = Initialize Array("" ("element"), w92) -> (w90:string[])
        n43 = call-poly <vilib>:"write multiple elements.vi"("values"=w90, "indices"=w93, "data table in"=w94) -> ("data table out"=w89:T3)  [unwired: 8 in]
      }
      frame "Boolean" {
        n44 = Array Size(array=w99) -> (size(s)=w98:i32)
        n45 = Initialize Array(FALSE, w98) -> (w96:bool[])
        n46 = call-poly <vilib>:"write multiple elements.vi"("values"=w96, "indices"=w99, "data table in"=w100) -> ("data table out"=w95:T3)  [unwired: 8 in]
      }
      frame Default {
      }
    }
  }
  n47 = Unbundle By Name(w12) -> ("output data.data table"=w11:T3)
  n48 = for {
    shift-right: [w104] -> w14
    shift-left: w5 -> [w104]
    shift-right: [w103] -> w13
    shift-left: w4 -> [w103]
    shift-right: [w102] -> _
    shift-left: w11 -> [w110]
    tunnel: w15 -> [w108] mode=indexing
    n49 = Unbundle By Name(w108) -> ("data type"=w106:T5, "indices"=w107:cluster{"index":i32[]})
    n50 = Wait Until Next ms Multiple(millisecond multiple=u32 100) -> ()  [unwired: 1 out]
    n51 = Unbundle(w107) -> ("index"=w105:i32[])
    n52 = case shown="\"Double\"" w106 {
      tunnel: w110 -> [w116 w122 w128 w134 w140 w146 w152 w158 w164 w170 w176 w182 w183]
      tunnel: [w111 w117 w123 w129 w135 w141 w147 w153 w159 w165 w171 w177 w183] -> w102
      tunnel: w105 -> [w115 w121 w127 w133 w139 w145 w151 w157 w163 w169 w175 w181 _]
      frame "Double" {
        n53 = Array Size(array=w115) -> (size(s)=w114:i32)
        n54 = Initialize Array(0.0 ("element"), w114) -> (w112:dbl[])
        n55 = call-poly <vilib>:"write multiple elements.vi"("values"=w112, "indices"=w115, "data table in"=w116) -> ("data table out"=w111:T3)  [unwired: 8 in]
      }
      frame "Single" {
        n56 = Array Size(array=w121) -> (size(s)=w120:i32)
        n57 = Initialize Array(sgl 0.0 ("element"), w120) -> (w118:sgl[])
        n58 = call-poly <vilib>:"write multiple elements.vi"("values"=w118, "indices"=w121, "data table in"=w122) -> ("data table out"=w117:T3)  [unwired: 8 in]
      }
      frame "I64" {
        n59 = Array Size(array=w127) -> (size(s)=w126:i32)
        n60 = Initialize Array(i64 0 ("element"), w126) -> (w124:i64[])
        n61 = call-poly <vilib>:"write multiple elements.vi"("values"=w124, "indices"=w127, "data table in"=w128) -> ("data table out"=w123:T3)  [unwired: 8 in]
      }
      frame "I32" {
        n62 = Array Size(array=w133) -> (size(s)=w132:i32)
        n63 = Initialize Array(0 ("element"), w132) -> (w130:i32[])
        n64 = call-poly <vilib>:"write multiple elements.vi"("values"=w130, "indices"=w133, "data table in"=w134) -> ("data table out"=w129:T3)  [unwired: 8 in]
      }
      frame "I16" {
        n65 = Array Size(array=w139) -> (size(s)=w138:i32)
        n66 = Initialize Array(i16 0 ("element"), w138) -> (w136:i16[])
        n67 = call-poly <vilib>:"write multiple elements.vi"("values"=w136, "indices"=w139, "data table in"=w140) -> ("data table out"=w135:T3)  [unwired: 8 in]
      }
      frame "I8" {
        n68 = Array Size(array=w145) -> (size(s)=w144:i32)
        n69 = Initialize Array(i8 0 ("element"), w144) -> (w142:i8[])
        n70 = call-poly <vilib>:"write multiple elements.vi"("values"=w142, "indices"=w145, "data table in"=w146) -> ("data table out"=w141:T3)  [unwired: 8 in]
      }
      frame "U64" {
        n71 = Array Size(array=w151) -> (size(s)=w150:i32)
        n72 = Initialize Array(u64 0 ("element"), w150) -> (w148:u64[])
        n73 = call-poly <vilib>:"write multiple elements.vi"("values"=w148, "indices"=w151, "data table in"=w152) -> ("data table out"=w147:T3)  [unwired: 8 in]
      }
      frame "U32" {
        n74 = Array Size(array=w157) -> (size(s)=w156:i32)
        n75 = Initialize Array(u32 0 ("element"), w156) -> (w154:u32[])
        n76 = call-poly <vilib>:"write multiple elements.vi"("values"=w154, "indices"=w157, "data table in"=w158) -> ("data table out"=w153:T3)  [unwired: 8 in]
      }
      frame "U16" {
        n77 = Array Size(array=w163) -> (size(s)=w162:i32)
        n78 = Initialize Array(u16 0 ("element"), w162) -> (w160:u16[])
        n79 = call-poly <vilib>:"write multiple elements.vi"("values"=w160, "indices"=w163, "data table in"=w164) -> ("data table out"=w159:T3)  [unwired: 8 in]
      }
      frame "U8" {
        n80 = Array Size(array=w169) -> (size(s)=w168:i32)
        n81 = Initialize Array(u8 0 ("element"), w168) -> (w166:u8[])
        n82 = call-poly <vilib>:"write multiple elements.vi"("values"=w166, "indices"=w169, "data table in"=w170) -> ("data table out"=w165:T3)  [unwired: 8 in]
      }
      frame "String" {
        n83 = Array Size(array=w175) -> (size(s)=w174:i32)
        n84 = Initialize Array("" ("element"), w174) -> (w172:string[])
        n85 = call-poly <vilib>:"write multiple elements.vi"("values"=w172, "indices"=w175, "data table in"=w176) -> ("data table out"=w171:T3)  [unwired: 8 in]
      }
      frame "Boolean" {
        n86 = Array Size(array=w181) -> (size(s)=w180:i32)
        n87 = Initialize Array(FALSE, w180) -> (w178:bool[])
        n88 = call-poly <vilib>:"write multiple elements.vi"("values"=w178, "indices"=w181, "data table in"=w182) -> ("data table out"=w177:T3)  [unwired: 8 in]
      }
      frame Default {
      }
    }
  }
  n89 = call-dynamic "close.vi"("error in"=w13, "shared memory module runtime"=w14) -> ("error out"=→"error out":errorcluster)  [unwired: 9 in]
